vi "fg_ROI Management.vi"(0 "Dwell Time [us]":dbl, 1 "ROIs for deletion":i32[](array[numeric]), 2 "Laser Power %":dbl, 3 "Function":T5, 5 "Offsets cluster":T2, 7 "XYZ":T1 {"Apparent Frame Size" format="%#_6f"; "Original FOV (um)" format="%#_6f"; "Pixels per miniscan" format="%#_6f"; "Dwell Time per pixel" format="%#_6f"; "Resolution" format="%#_6f"; "ROI group ID" format="%#_6f"; "Laser Power (%)" format="%#_6f"; "Zoom" format="%#_6f"; "Frame Size" format="%#_6f"; "Number of lines" format="%#_6f"; "Composite ID" format="%#_6f"; "Angle (deg)" format="%#_6f"; "ROI Time (ns)" format="%#_6f"; "ROI ID" format="%#_6f"; "Pixels in ROI" format="%#_6f"; "ROI index" format="%#_6f"; "Z stop" format="%#_6f"; "Y stop" format="%#_6f"; "X stop" format="%#_6f"; "Z start" format="%#_6f"; "X start" format="%#_6f"; "Y start" format="%#_6f"}, 9 "ROI management Input cluster":T3, 11 "error in (no error)":errorcluster, 13 "ROI Setup Array Idx to modify":i32) -> (4 "ROI Setup":T1[](array[typedef]) {"Apparent Frame Size" format="%#_6f"; "Original FOV (um)" format="%#_6f"; "Pixels per miniscan" format="%#_6f"; "Dwell Time per pixel" format="%#_6f"; "Resolution" format="%#_6f"; "ROI group ID" format="%#_6f"; "Laser Power (%)" format="%#_6f"; "Zoom" format="%#_6f"; "Frame Size" format="%#_6f"; "Number of lines" format="%#_6f"; "Composite ID" format="%#_6f"; "Angle (deg)" format="%#_6f"; "ROI Time (ns)" format="%#_6f"; "ROI ID" format="%#_6f"; "Pixels in ROI" format="%#_6f"; "ROI index" format="%#_6f"; "Z stop" format="%#_6f"; "Y stop" format="%#_6f"; "X stop" format="%#_6f"; "Z start" format="%#_6f"; "X start" format="%#_6f"; "Y start" format="%#_6f"}, 6 "Number of ROI":i32, 8 "Total ROI time":dbl, 10 "Last composite ID":i32, 12 "Exceeded limit number of lines":bool, 14 "No lines left":bool, 15 "error out":errorcluster)   [LabVIEW 2020]
uses:
  Visualisation/Functional Imaging Viewer/Typedefs/ROI parameters data type.ctl
  Typedefs/ROI management FG states.ctl
  Typedefs/ROI management Input cluster.ctl
  Typedefs/ROI ID Enum.ctl
  Typedefs/Offsets cluster.ctl
  Global Variables/General Globals.vi
  ROI Entry screen/Globals/gl_ROI Entry UI globals.vi
panel:
  out "Number of lines left":i32
  in  "Reuse last composite ID":bool
  # "[zero based]"
  # "X Start\nY Start\nX Stop\nY Stop"
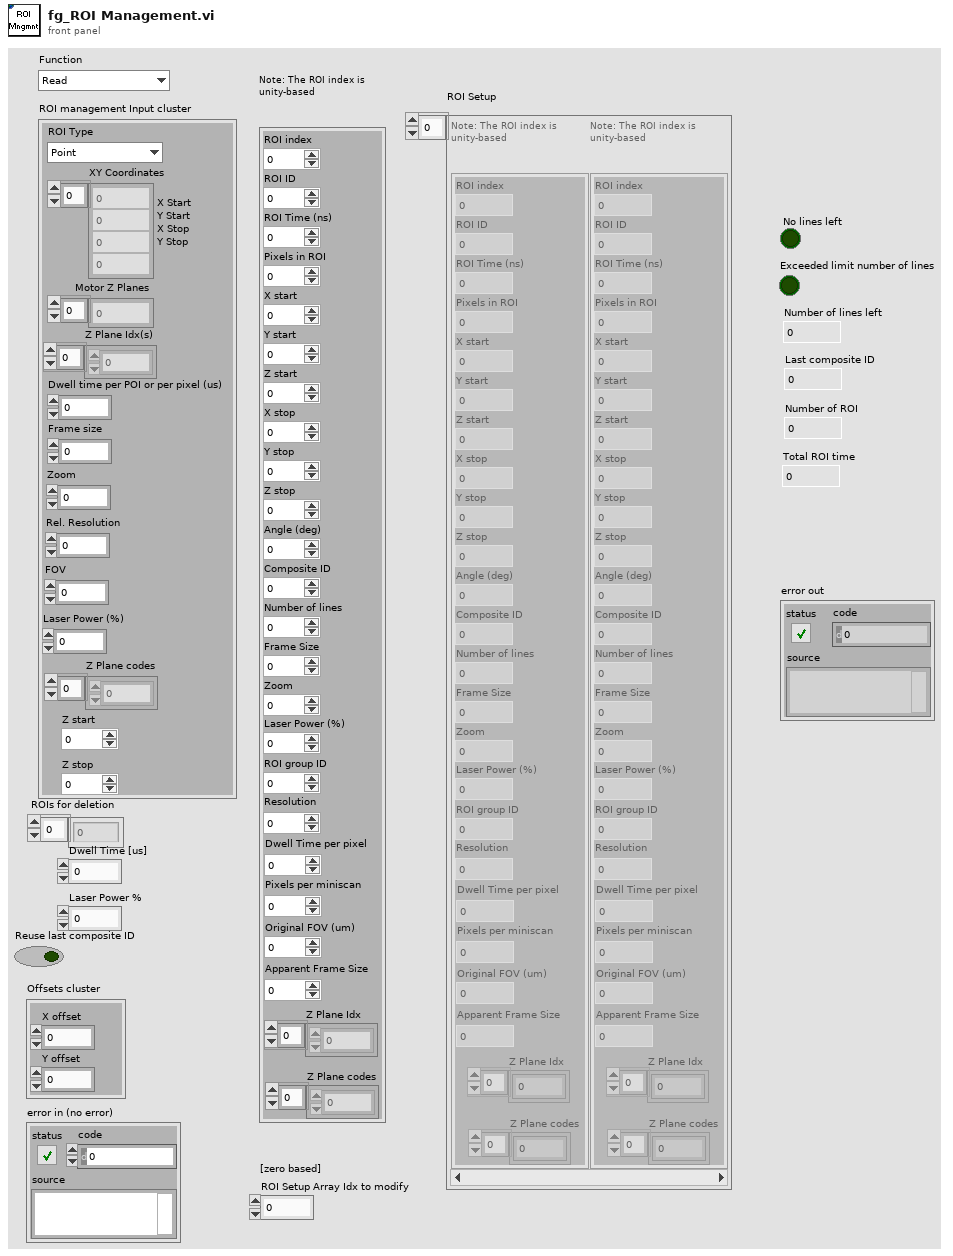
[diagram p1: front panel]
types:
  T1 = typedef "ROI parameters data type.ctl" = cluster{"ROI index":dbl, "ROI ID":dbl, "ROI Time (ns)":dbl, "Pixels in ROI":dbl, "X start":dbl, "Y start":dbl, "Z start":dbl, "X stop":dbl, "Y stop":dbl, "Z stop":dbl, "Angle (deg)":dbl, "Composite ID":dbl, "Number of lines":dbl, "Frame Size":dbl, "Zoom":dbl, "Laser Power (%)":dbl, "ROI group ID":dbl, "Resolution":dbl, "Dwell Time per pixel":dbl, "Pixels per miniscan":dbl, "Original FOV (um)":dbl, "Apparent Frame Size":dbl, "Z Plane Idx":i32[], "Z Plane codes":i32[]}
  T2 = typedef "Offsets cluster.ctl" = cluster{"X offset":i8, "Y offset":i8}
  T3 = typedef "ROI management Input cluster.ctl" = cluster{"ROI Type":T4, "XY Coordinates":i32[], "Motor Z Planes":dbl[], "Dwell time per POI or per pixel (us)":dbl, "Frame size":i32, "Zoom":dbl, "Rel. Resolution":dbl, "FOV":dbl, "Laser Power (%)":dbl, "Z Plane codes":u8[], "Z start":dbl, "Z stop":dbl, "Z Plane Idx(s)":i32[]}
  T4 = typedef "ROI ID Enum.ctl" = enum16{"Point", "MiniScan", "Comp. MiniScan", "Rectangle", "Comp. volume", "Arb. plane point", "None"}
  T5 = typedef "ROI management FG states.ctl" = enum16{"Read", "Write", "Write-from dataset", "Clear Last", "Clear All", "Delete ROI", "Update ROIs time", "Reload last ROI set", "Modify ROI Parameters", "Offset all ROI", "Offset visible ROI", "Modify Dwell Time", "Modify Laser Power"}
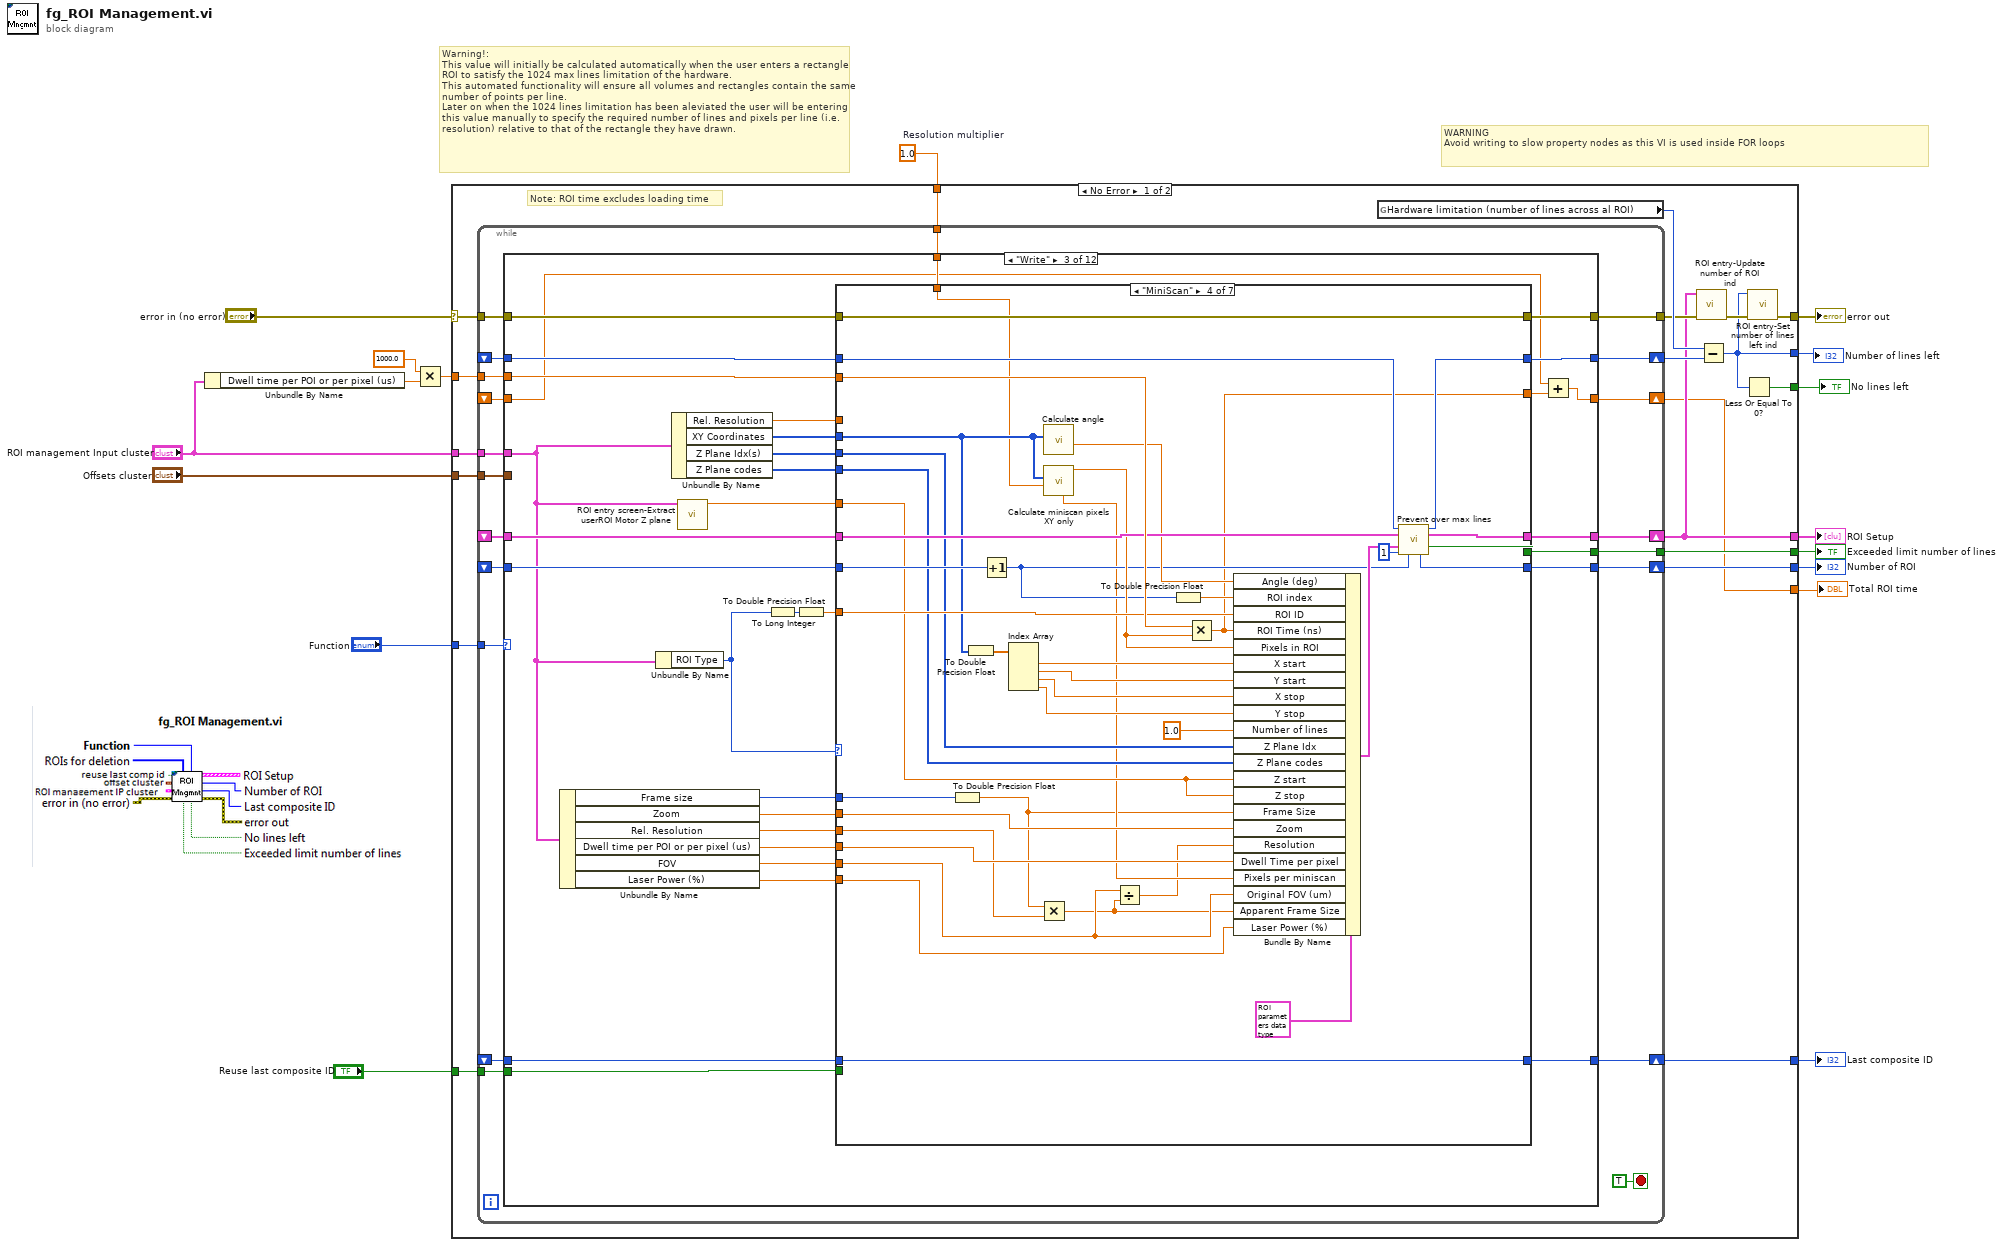
[diagram p0: block diagram]
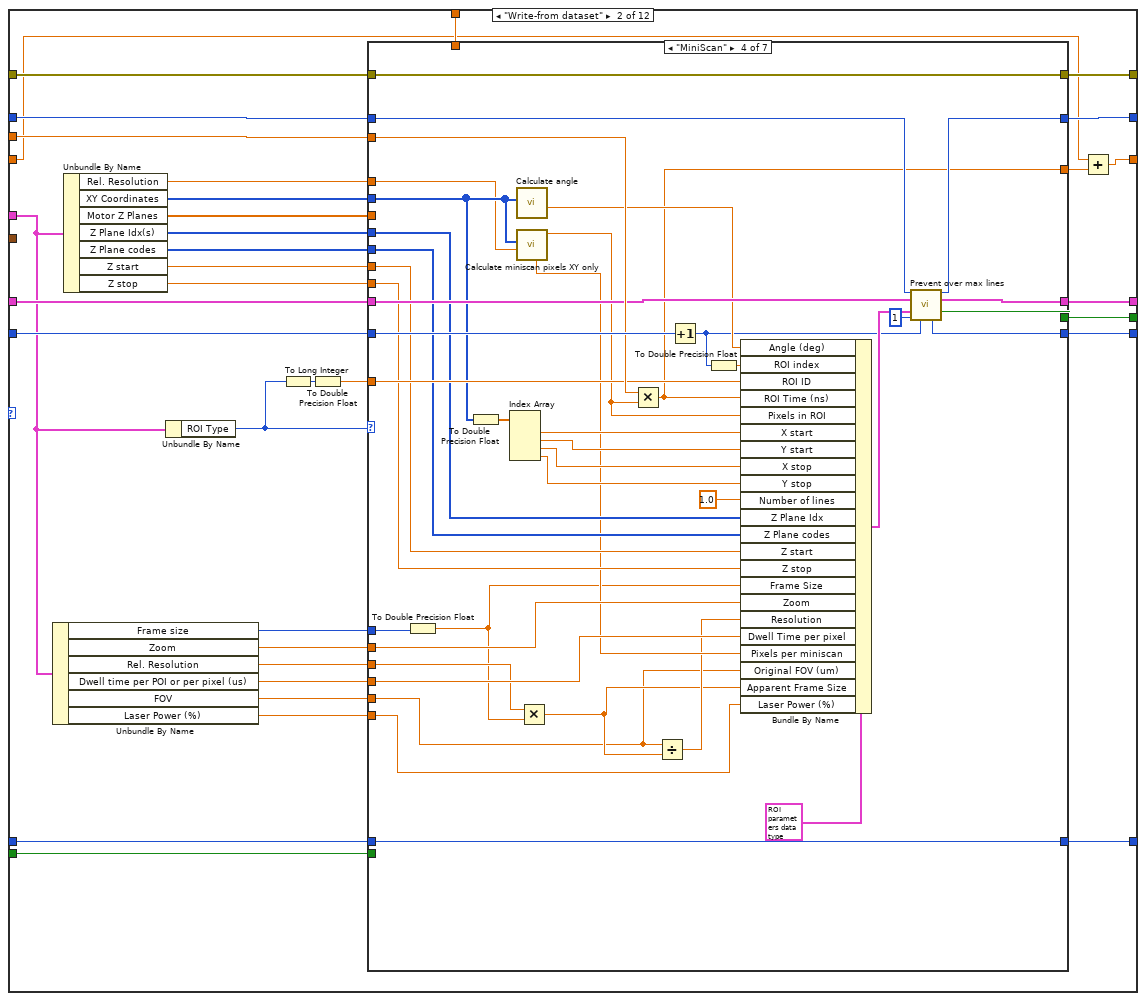
[diagram p3: hidden frame]
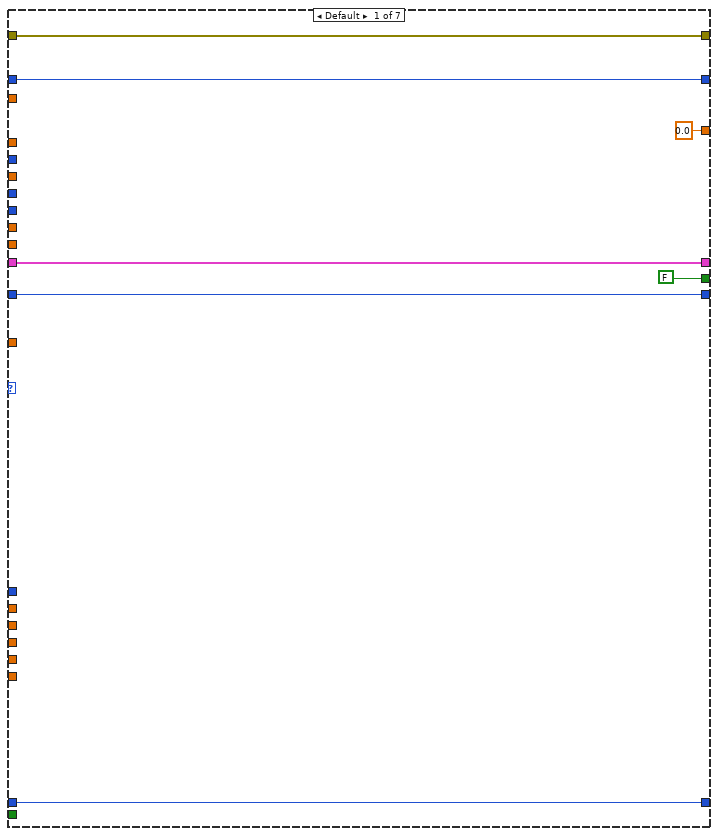
[diagram p4: hidden frame]
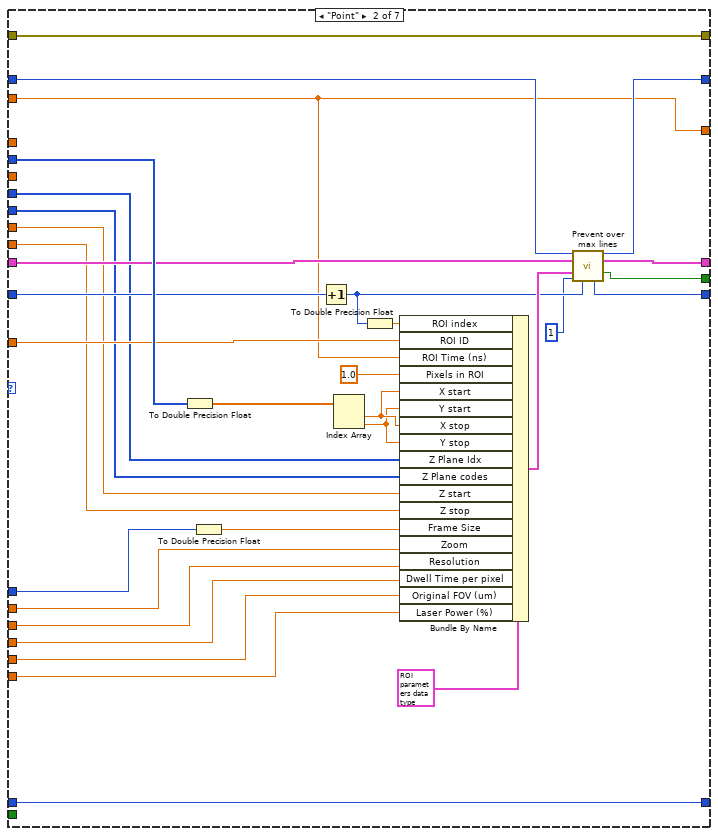
[diagram p5: hidden frame]
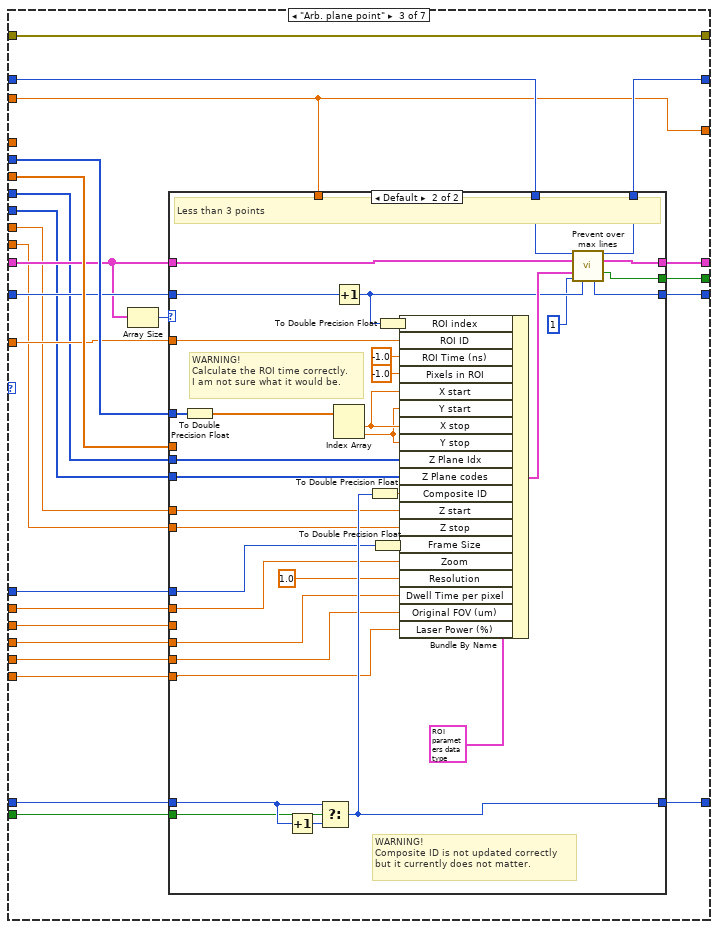
[diagram p6: hidden frame]
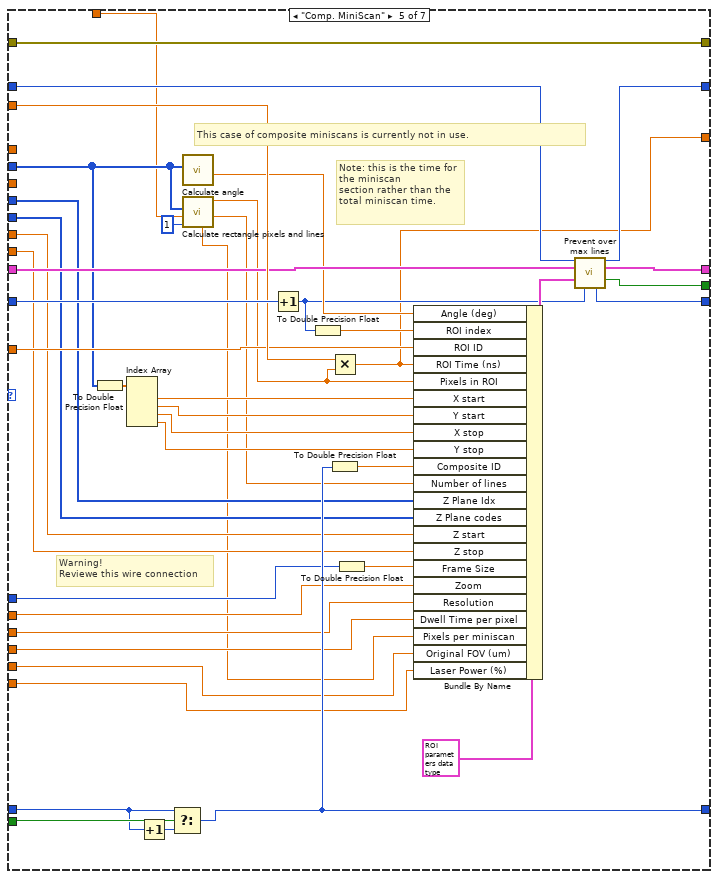
[diagram p8: hidden frame]
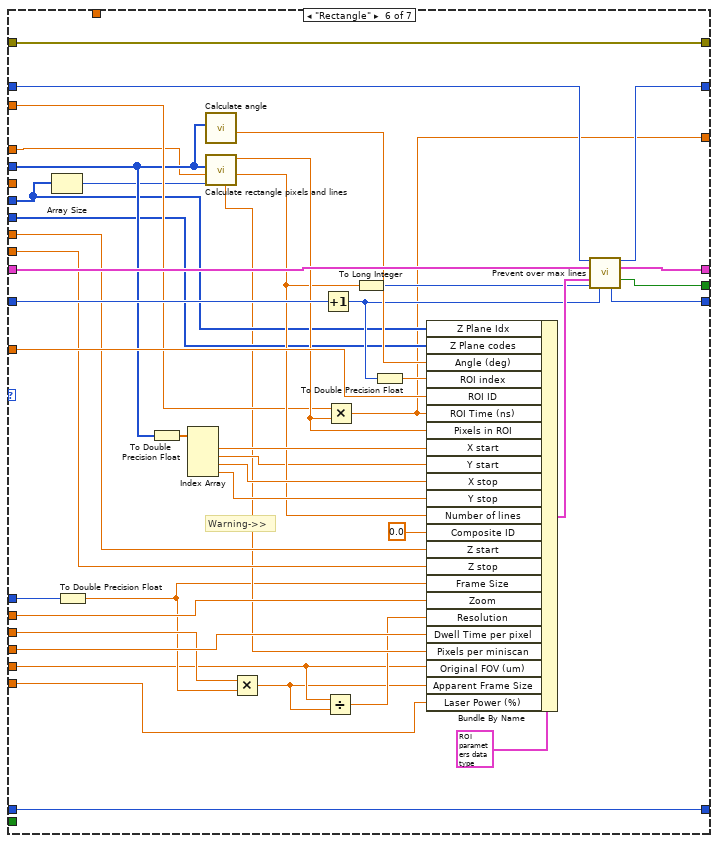
[diagram p9: hidden frame]
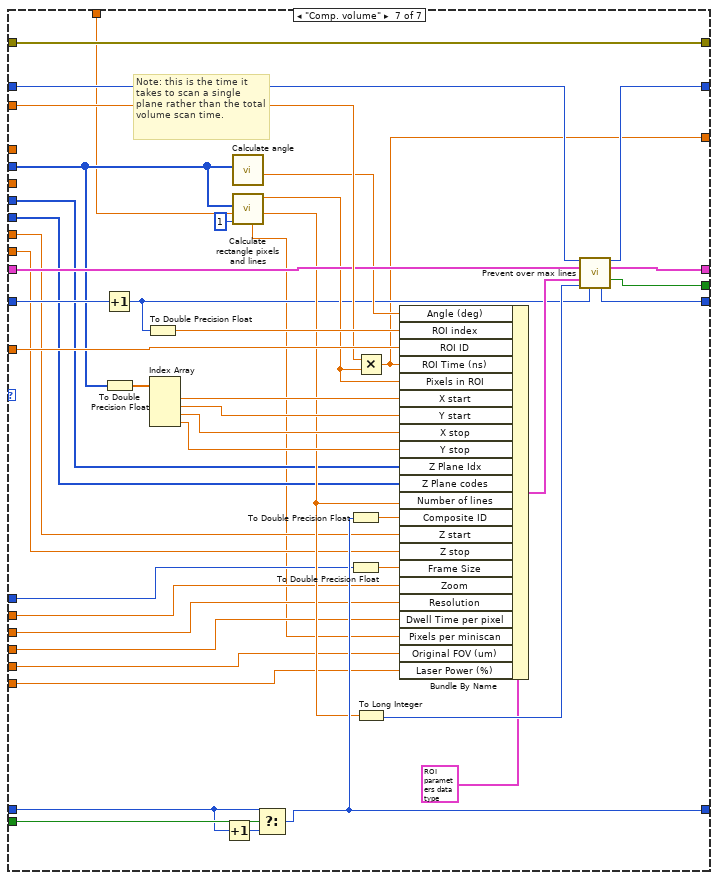
[diagram p10: hidden frame]
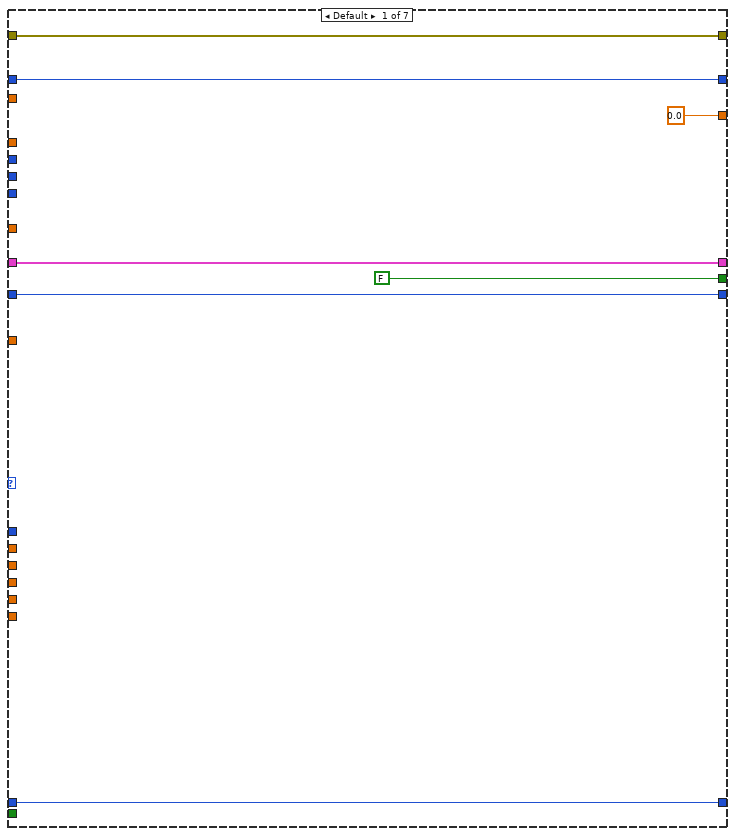
[diagram p11: hidden frame]
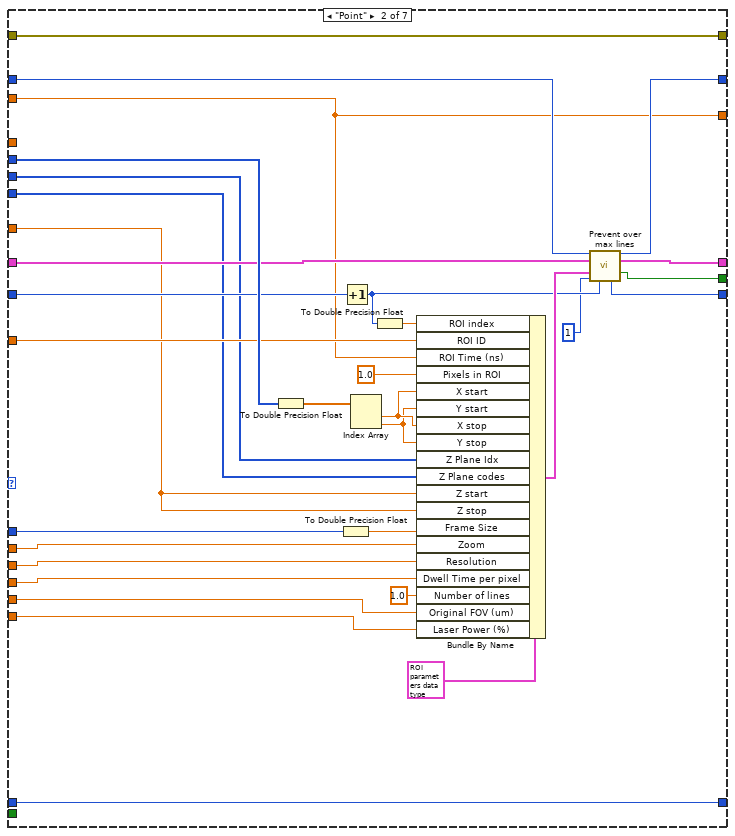
[diagram p12: hidden frame]
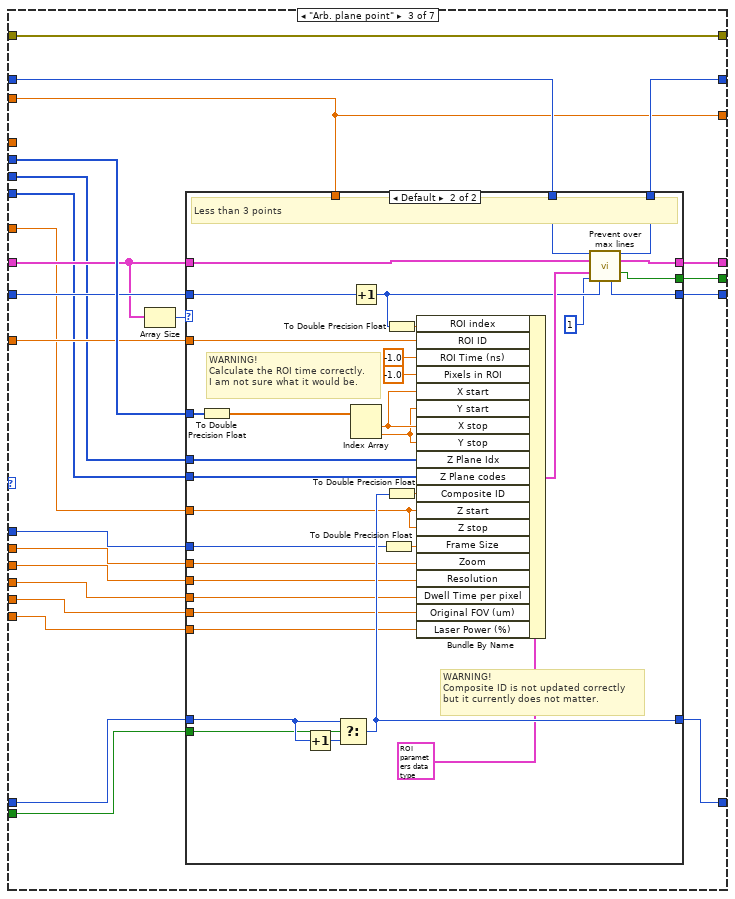
[diagram p13: hidden frame]
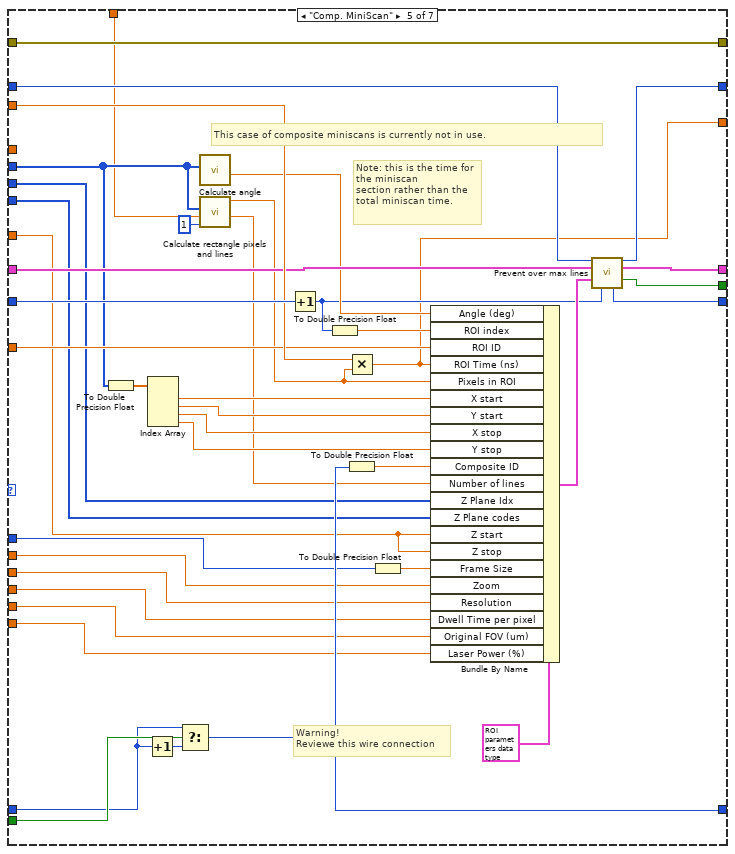
[diagram p15: hidden frame]
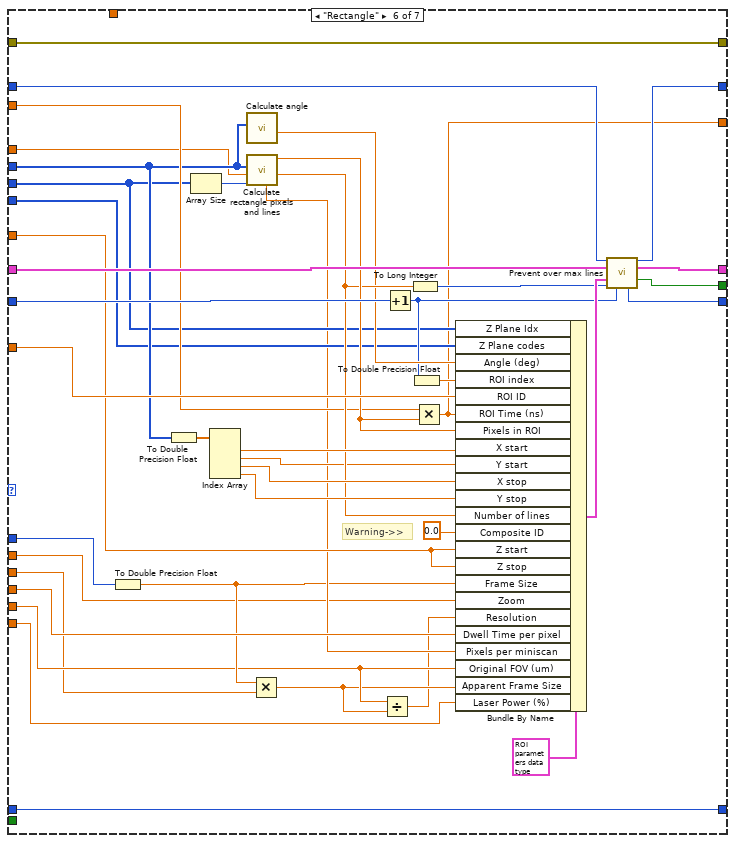
[diagram p16: hidden frame]
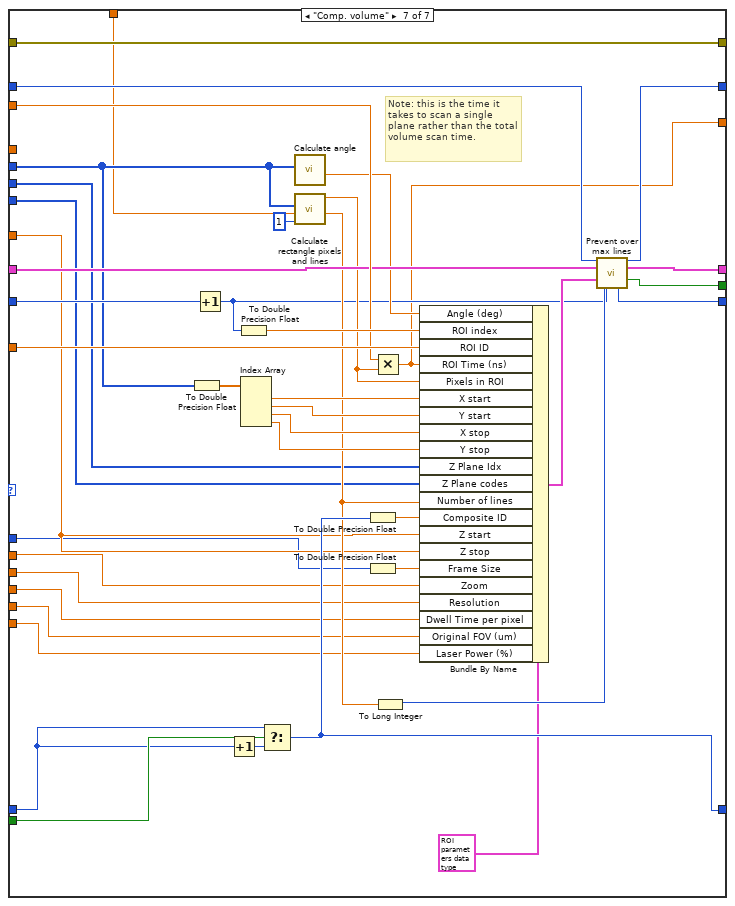
[diagram p17: hidden frame]
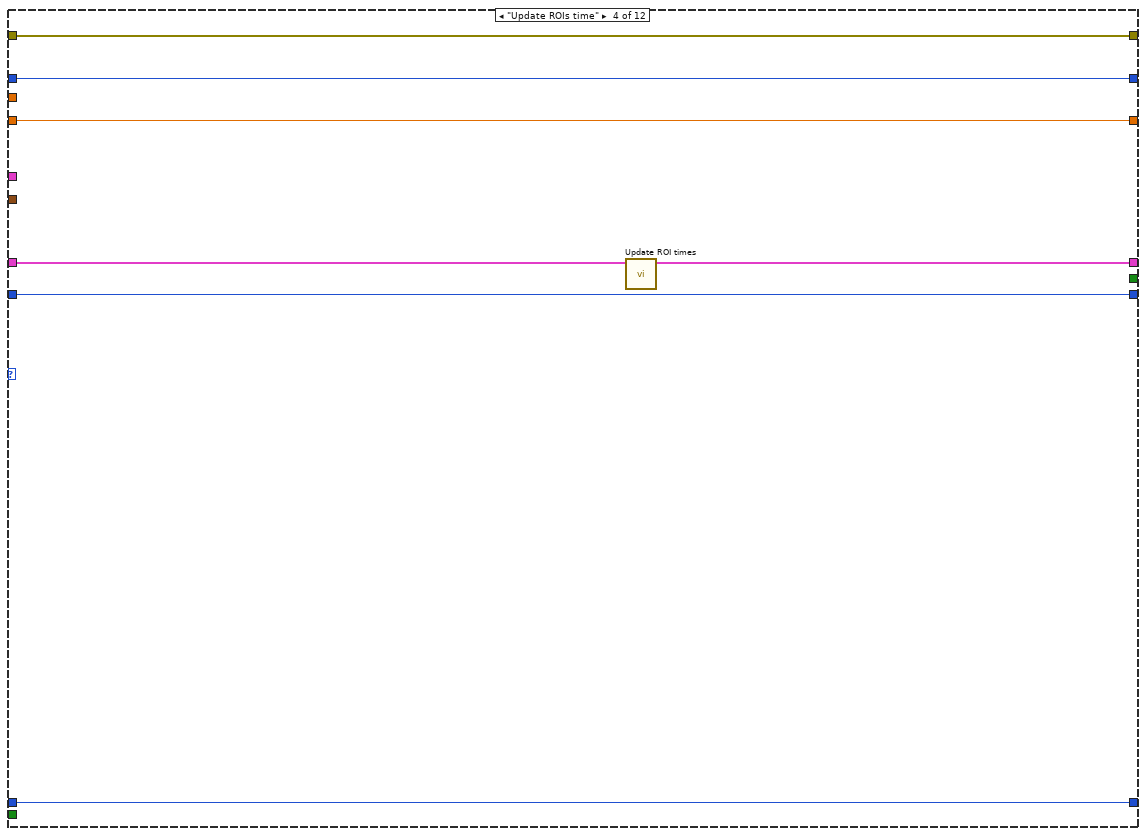
[diagram p18: hidden frame]
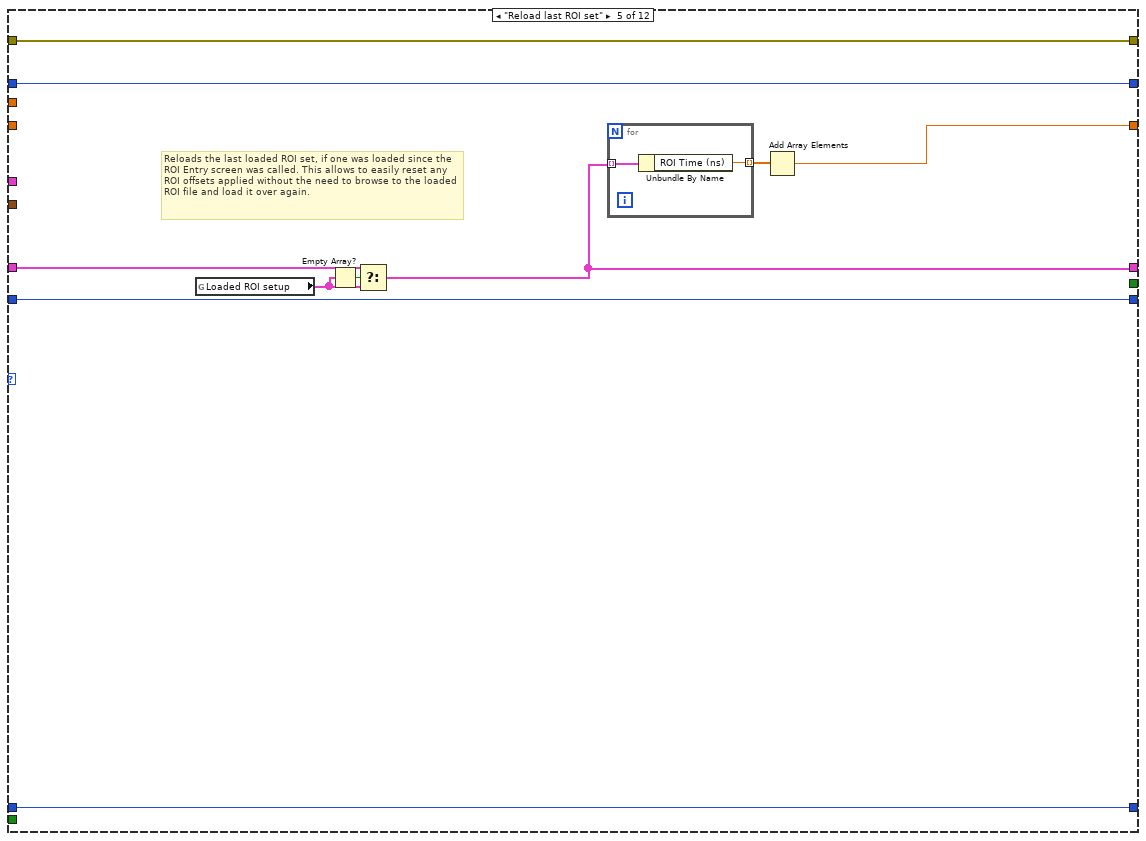
[diagram p19: hidden frame]
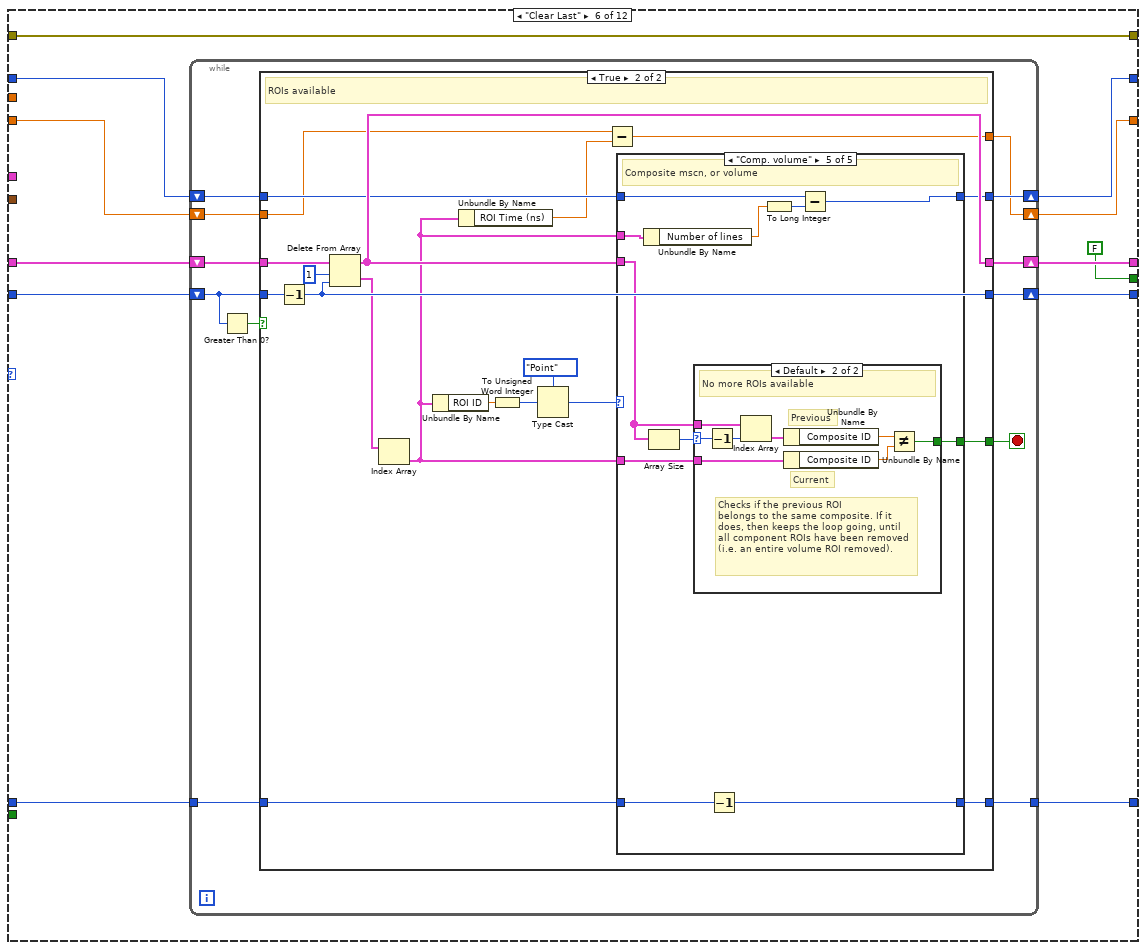
[diagram p20: hidden frame]
diagram:
  w7 = 1.0  # Resolution multiplier
  # "WARNING\nAvoid writing to slow property nodes as this VI is used inside FOR loops"
  # "Warning!:\nThis value will initially be calculated automatically when the user enters a rectangle ROI to satisfy the 1024 max lines limitation of the hardware.\nThis automated functionality will ensure all volumes and rectangles contain the same number of points per line.\nLater on when the 1024 lines limitation has been aleviated the user will be entering this value manually to specify the required number of lines and pixels per line (i.e. resolution) relative to that of the rectangle they have drawn."
  n1 = Unbundle By Name("ROI management Input cluster") -> ("Dwell time per POI or per pixel (us)"=w8:dbl)
  n2 = Multiply(x=1000.0, y=w8) -> (x*y=w13:dbl)
  n3 = case shown="No Error" "error in (no error)" {
    selector: "error in (no error)" -> [w36 w867]
    tunnel: [w22 w867] -> w14
    tunnel: [w24 _] -> w16
    tunnel: w13 -> [w35 _]
    tunnel: "Function" -> [w34 _]
    tunnel: [w33 _] -> w11
    tunnel: [w32 _] -> w10
    tunnel: "Reuse last composite ID" -> [w31 _]
    tunnel: "ROI management Input cluster" -> [w30 _]
    tunnel: w7 -> [w29 _]
    tunnel: [w20 _] -> w5
    tunnel: [w26 _] -> w4
    tunnel: "Offsets cluster" -> [w21 _]
    tunnel: [w19 _] -> w2
    tunnel: [w18 0.0 ("ROI Time (ns)o/p")] -> w1
    frame No Error {
      # "Note: ROI time excludes loading time"
      n4 = while {
        tunnel: w36 -> [w56]
        tunnel: [w55] -> w25
        shift-right: [w54] -> w24
        shift-left: _ -> [w52]
        tunnel: w35 -> [w53]
        shift-right: [w51] -> w33
        shift-left: _ -> [w50]
        tunnel: w34 -> [w49]
        shift-right: [w46] -> w32
        shift-left: _ -> [w47]
        tunnel: w31 -> [w45]
        tunnel: w30 -> [w44]
        shift-right: [w43] -> w28
        shift-left: _ -> [w42]
        tunnel: w29 -> [w41]
        tunnel: [w40] -> w26
        tunnel: w21 -> [w39]
        shift-right: [w38] -> w18
        shift-left: _ -> [w37]
        stop <- TRUE stop-if-true
        n5 = case shown="\"Write\"" w49 {
          selector: w49 -> [_ _ _ _ _ _ _ w798 _ _ _ _]
          tunnel: w56 -> [w60 w96 w403 w674 w685 w698 w795 w804 w809 w831 w842 w858]
          tunnel: [w60 w95 w402 w674 w685 w698 w795 w804 w809 w831 w842 w858] -> w55
          tunnel: [w62 w94 w401 w676 w679 w699 T1[] [] w799 w814 w825 w845 w860] -> w54
          tunnel: w53 -> [_ w93 w373 _ _ _ _ _ _ _ _ _]
          tunnel: w52 -> [w62 w92 w400 w672 w681 w694 _ w802 w815 w817 w847 w862]
          tunnel: [w61 w91 w399 w675 w686 w700 0 w805 w813 w818 w844 w859] -> w51
          tunnel: w50 -> [w61 w90 w398 w675 w686 w695 _ w805 _ w819 w844 w859]
          tunnel: w47 -> [w59 w86 w394 w671 w683 w697 _ w801 w808 w830 w841 w856]
          tunnel: [w59 w87 w395 w671 w683 w696 0 ("Last composite ID") w801 w808 w830 w841 w856] -> w46
          tunnel: w45 -> [_ w85 w393 _ _ _ _ _ _ _ _ _]
          tunnel: w44 -> [_ w81 w384 _ _ _ _ _ _ _ _ _]
          tunnel: [w58 w78 w388 w673 w684 w691 0 w803 w810 w820 w843 w857] -> w43
          tunnel: w42 -> [w58 w80 w390 w673 w684 w693 _ w803 w811 w821 w843 w857]
          tunnel: w41 -> [_ w79 w389 _ _ _ _ _ _ _ _ _]
          tunnel: [_ w77 w387 _ _ FALSE ("Exceeded 1024 lines") FALSE ("Exceeded 1024 lines") _ _ _ _ _] -> w40
          tunnel: w39 -> [_ _ _ _ _ _ _ w800 _ _ _ _]
          tunnel: [w57 w63 w375 w670 w677 w689 0.0 w797 w806 w826 w839 w855] -> w38
          tunnel: w37 -> [w57 w65 w372 w670 _ w690 _ w797 w807 w828 _ w855]
          frame "Read", Default {
          }
          frame "Write-from dataset" {
            n6 = Unbundle By Name(w81) -> ("Frame size"=w72:i32, "Zoom"=w71:dbl, "Rel. Resolution"=w70:dbl, "Dwell time per POI or per pixel (us)"=w69:dbl, "FOV"=w67:dbl, "Laser Power (%)"=w66:dbl)
            n7 = Unbundle By Name(w81) -> ("Rel. Resolution"=w68:dbl, "XY Coordinates"=w84:i32[], "Motor Z Planes"=w83:dbl[], "Z Plane Idx(s)"=w76:i32[], "Z Plane codes"=w75:u8[], "Z start"=w74:dbl, "Z stop"=w73:dbl)
            n8 = Unbundle By Name(w81) -> ("ROI Type"=w82:T4)
            n9 = To Long Integer(number=w82) -> (32bit integer=w89:i32)
            n10 = To Double Precision Float(number=w89) -> (double precision float=w88:dbl)
            n11 = case shown="\"MiniScan\"" w82 {
              tunnel: w84 -> [_ w134 w159 w225 w263 w308 w349]
              tunnel: w83 -> [_ _ w160 _ _ _ _]
              tunnel: w96 -> [w101 w135 w161 w241 w284 w327 w371]
              tunnel: [w101 w135 w161 w241 w284 w327 w371] -> w95
              tunnel: [w103 w125 w157 w229 w267 w319 w354] -> w94
              tunnel: w93 -> [_ w104 w136 w237 w280 w309 w362]
              tunnel: w92 -> [w103 w126 w153 w231 w269 w321 w356]
              tunnel: w90 -> [w102 w132 w158 w240 w283 w326 w370]
              tunnel: [w102 w119 w151 w220 w257 w303 w343] -> w91
              tunnel: w88 -> [_ w128 w147 w234 w275 w324 w364]
              tunnel: [w100 w127 w148 w233 w271 w322 w357] -> w87
              tunnel: w86 -> [w100 w127 w150 w233 w270 w322 w359]
              tunnel: w85 -> [_ _ w149 _ w272 _ w360]
              tunnel: [w99 w124 w156 w227 w266 w318 w353] -> w78
              tunnel: w80 -> [w99 w123 w155 w228 w265 w317 w352]
              tunnel: w79 -> [_ _ _ _ w260 _ w345]
              tunnel: [FALSE ("Exceeded 1024 lines") w122 w154 w226 w264 w316 w350] -> w77
              tunnel: w76 -> [_ w117 w146 w218 w255 w301 w341]
              tunnel: w75 -> [_ w118 w145 w219 w256 w302 w342]
              tunnel: w74 -> [_ w115 w144 w217 w254 w299 w339]
              tunnel: w73 -> [_ w114 w143 w216 w253 w298 w338]
              tunnel: w72 -> [_ w112 w142 w213 w250 w291 w336]
              tunnel: w71 -> [_ w111 w141 w212 w249 w297 w335]
              tunnel: w70 -> [_ w110 w140 w207 w248 w292 w334]
              tunnel: w69 -> [_ w109 w139 w211 w247 w296 w333]
              tunnel: w68 -> [_ _ _ w208 _ w293 _]
              tunnel: w67 -> [_ w107 w138 w203 w244 w288 w330]
              tunnel: w66 -> [_ w106 w137 w202 w243 w286 w329]
              tunnel: [0.0 w104 w136 w201 w242 w285 w328] -> w64
              frame Default {
              }
              frame "Point" {
                n12 = To Double Precision Float(number=w134) -> (double precision float=w130:dbl[])
                n13 = To Double Precision Float(number=w112) -> (double precision float=w113:dbl)
                n14 = Increment(x=w132) -> (x+1=w120:i32)
                n15 = Index Array(array=w130) -> (element #1=w131:dbl, element #2=w121:dbl)  [unwired: 2 in]
                n16 = To Double Precision Float(number=w120) -> (double precision float=w129:dbl)
                n17 = Bundle By Name(cluster=T1 {"ROI index"=0.0, "ROI ID"=0.0, "ROI Time (ns)"=0.0, "Pixels in ROI"=0.0, "X start"=0.0, "Y start"=0.0, "Z start"=0.0, "X stop"=0.0, "Y stop"=0.0, "Z stop"=0.0, "Angle (deg)"=0.0, "Composite ID"=0.0, "Number of lines"=0.0, "Frame Size"=0.0, "Zoom"=0.0, "Laser Power (%)"=0.0, "ROI group ID"=0.0, "Resolution"=0.0, "Dwell Time per pixel"=0.0, "Pixels per miniscan"=0.0, "Original FOV (um)"=0.0, "Apparent Frame Size"=0.0, "Z Plane Idx"=[], "Z Plane codes"=[]} ("X-Y-Z coordinates"), "ROI index"=w129, "ROI ID"=w128, "ROI Time (ns)"=w104, "Pixels in ROI"=1.0 ("#Pixels"), "X start"=w131, "Y start"=w121, "X stop"=w131, "Y stop"=w121, "Z Plane Idx"=w117, "Z Plane codes"=w118, "Z start"=w115, "Z stop"=w114, "Frame Size"=w113, "Zoom"=w111, "Resolution"=w110, "Dwell Time per pixel"=w109, "Original FOV (um)"=w107, "Laser Power (%)"=w106) -> (w133:T1)
                n18 = call "Prevent over max lines.vi"("Existing number of lines across all ROI"=w123, "Array in"=w126, "X-Y-Z coordinates"=w133, "New number of lines to be added (1)"=1, "Number of ROI"=w120) -> ("Resulting number of lines across all ROI"=w124:i32, "Array out"=w125:T1[], "Exceeded 1024 lines"=w122:bool, "Number of ROI"=w119:i32)  [unwired: 5 in, 2 out]
              }
              frame "Arb. plane point" {
                n19 = Array Size(array=w153) -> (size(s)=w152:i32)
                n20 = case shown="Default" w152 {
                  selector: w152 -> [w163 _]
                  tunnel: w160 -> [_ _]
                  tunnel: w159 -> [_ w200]
                  tunnel: w158 -> [_ w198]
                  tunnel: w136 -> [_ _]
                  tunnel: [w164 w193] -> w157
                  tunnel: [w165 w192] -> w156
                  tunnel: w155 -> [w165 w191]
                  tunnel: [_ w190] -> w154
                  tunnel: w153 -> [w164 w188]
                  tunnel: [w163 w179] -> w151
                  tunnel: w150 -> [w162 w186]
                  tunnel: w149 -> [_ w185]
                  tunnel: [w162 w183] -> w148
                  tunnel: w147 -> [_ w182]
                  tunnel: w146 -> [_ w177]
                  tunnel: w145 -> [_ w178]
                  tunnel: w144 -> [_ w175]
                  tunnel: w143 -> [_ w174]
                  tunnel: w142 -> [_ w171]
                  tunnel: w141 -> [_ w170]
                  tunnel: w140 -> [_ _]
                  tunnel: w139 -> [_ w169]
                  tunnel: w138 -> [_ w167]
                  tunnel: w137 -> [_ w166]
                  frame 3.. {
                    # "3 points (or more) already entered"
                  }
                  frame Default {
                    # "WARNING!\nComposite ID is not updated correctly\nbut it currently does not matter."
                    # "WARNING!\nCalculate the ROI time correctly.\nI am not sure what it would be."
                    # "Less than 3 points"
                    n21 = To Double Precision Float(number=w200) -> (double precision float=w195:dbl[])
                    n22 = Increment(x=w186) -> (x+1=w187:i32)
                    n23 = Select(t=w186, s=w185, f=w187) -> (s? t:f=w183:i32)
                    n24 = Increment(x=w198) -> (x+1=w180:i32)
                    n25 = Index Array(array=w195) -> (element #1=w196:dbl, element #2=w189:dbl)  [unwired: 2 in]
                    n26 = To Double Precision Float(number=w183) -> (double precision float=w184:dbl)
                    n27 = To Double Precision Float(number=w171) -> (double precision float=w172:dbl)
                    n28 = To Double Precision Float(number=w180) -> (double precision float=w194:dbl)
                    n29 = Bundle By Name(cluster=T1 {"ROI index"=0.0, "ROI ID"=0.0, "ROI Time (ns)"=0.0, "Pixels in ROI"=0.0, "X start"=0.0, "Y start"=0.0, "Z start"=0.0, "X stop"=0.0, "Y stop"=0.0, "Z stop"=0.0, "Angle (deg)"=0.0, "Composite ID"=0.0, "Number of lines"=0.0, "Frame Size"=0.0, "Zoom"=0.0, "Laser Power (%)"=0.0, "ROI group ID"=0.0, "Resolution"=0.0, "Dwell Time per pixel"=0.0, "Pixels per miniscan"=0.0, "Original FOV (um)"=0.0, "Apparent Frame Size"=0.0, "Z Plane Idx"=[], "Z Plane codes"=[]} ("X-Y-Z coordinates"), "ROI index"=w194, "ROI ID"=w182, "ROI Time (ns)"=-1.0, "Pixels in ROI"=-1.0 ("#Pixels"), "X start"=w196, "Y start"=w189, "X stop"=w196, "Y stop"=w189, "Z Plane Idx"=w177, "Z Plane codes"=w178, "Composite ID"=w184, "Z start"=w175, "Z stop"=w174, "Frame Size"=w172, "Zoom"=w170, "Resolution"=1.0, "Dwell Time per pixel"=w169, "Original FOV (um)"=w167, "Laser Power (%)"=w166) -> (w199:T1)
                    n30 = call "Prevent over max lines.vi"("Existing number of lines across all ROI"=w191, "Array in"=w188, "X-Y-Z coordinates"=w199, "New number of lines to be added (1)"=1, "Number of ROI"=w180) -> ("Resulting number of lines across all ROI"=w192:i32, "Array out"=w193:T1[], "Exceeded 1024 lines"=w190:bool, "Number of ROI"=w179:i32)  [unwired: 5 in, 2 out]
                  }
                }
              }
              frame "MiniScan" {
                n31 = To Double Precision Float(number=w213) -> (double precision float=w206:dbl)
                n32 = To Double Precision Float(number=w225) -> (double precision float=w238:dbl[])
                n33 = Index Array(array=w238) -> (element #1=w222:dbl, element #2=w239:dbl, element #3=w232:dbl, element #4=w235:dbl)  [unwired: 4 in]
                n34 = call "Calculate angle.vi"("XY Coordinates"=w225) -> ("Angle (deg)"=w223:dbl)  [unwired: 10 in]
                n35 = call "Calculate miniscan pixels XY only.vi"("Resolution multiplier"=w208, "XY Coordinates (zero based)"=w225) -> ("Pixels in ROI"=w224:dbl, "X pixels"=w209:dbl)  [unwired: 7 in, 1 out]
                n36 = Multiply(x=w207, y=w206) -> (x*y=w204:dbl)
                n37 = Multiply(x=w237, y=w224) -> (x*y=w201:dbl)
                n38 = Divide(x=w203, y=w204) -> (x/y=w205:dbl)
                n39 = Increment(x=w240) -> (x+1=w221:i32)
                n40 = To Double Precision Float(number=w221) -> (double precision float=w236:dbl)
                n41 = Bundle By Name(cluster=T1 {"ROI index"=0.0, "ROI ID"=0.0, "ROI Time (ns)"=0.0, "Pixels in ROI"=0.0, "X start"=0.0, "Y start"=0.0, "Z start"=0.0, "X stop"=0.0, "Y stop"=0.0, "Z stop"=0.0, "Angle (deg)"=0.0, "Composite ID"=0.0, "Number of lines"=0.0, "Frame Size"=0.0, "Zoom"=0.0, "Laser Power (%)"=0.0, "ROI group ID"=0.0, "Resolution"=0.0, "Dwell Time per pixel"=0.0, "Pixels per miniscan"=0.0, "Original FOV (um)"=0.0, "Apparent Frame Size"=0.0, "Z Plane Idx"=[], "Z Plane codes"=[]} ("X-Y-Z coordinates"), "Angle (deg)"=w223, "ROI index"=w236, "ROI ID"=w234, "ROI Time (ns)"=w201, "Pixels in ROI"=w224, "X start"=w222, "Y start"=w239, "X stop"=w232, "Y stop"=w235, "Number of lines"=1.0, "Z Plane Idx"=w218, "Z Plane codes"=w219, "Z start"=w217, "Z stop"=w216, "Frame Size"=w206, "Zoom"=w212, "Resolution"=w205, "Dwell Time per pixel"=w211, "Pixels per miniscan"=w209, "Original FOV (um)"=w203, "Apparent Frame Size"=w204, "Laser Power (%)"=w202) -> (w230:T1)
                n42 = call "Prevent over max lines.vi"("Existing number of lines across all ROI"=w228, "Array in"=w231, "X-Y-Z coordinates"=w230, "New number of lines to be added (1)"=1, "Number of ROI"=w221) -> ("Resulting number of lines across all ROI"=w227:i32, "Array out"=w229:T1[], "Exceeded 1024 lines"=w226:bool, "Number of ROI"=w220:i32)  [unwired: 5 in, 2 out]
              }
              frame "Comp. MiniScan" {
                # "This case of composite miniscans is currently not in use."
                # "Warning!\nReviewe this wire connection"
                # "Note: this is the time for the miniscan\nsection rather than the total miniscan time."
                n43 = To Double Precision Float(number=w263) -> (double precision float=w281:dbl[])
                n44 = Index Array(array=w281) -> (element #1=w278:dbl, element #2=w282:dbl, element #3=w277:dbl, element #4=w276:dbl)  [unwired: 4 in]
                n45 = Increment(x=w270) -> (x+1=w273:i32)
                n46 = Select(t=w270, s=w272, f=w273) -> (s? t:f=w271:i32)
                n47 = call "Calculate angle.vi"("XY Coordinates"=w263) -> ("Angle (deg)"=w261:dbl)  [unwired: 10 in]
                n48 = call "Calculate rectangle pixels and lines.vi"("No of Z planes"=1, "Resolution multiplier"=w260, "XY Coordinates (zero based)"=w263) -> ("Number of lines (scaled)"=w259:dbl, "Pixels in ROI"=w262:dbl, "X pixels"=w245:dbl)  [unwired: 6 in]
                n49 = Increment(x=w283) -> (x+1=w258:i32)
                n50 = To Double Precision Float(number=w258) -> (double precision float=w279:dbl)
                n51 = Multiply(x=w280, y=w262) -> (x*y=w242:dbl)
                n52 = To Double Precision Float(number=w271) -> (double precision float=w274:dbl)
                n53 = To Double Precision Float(number=w250) -> (double precision float=w251:dbl)
                n54 = Bundle By Name(cluster=T1 {"ROI index"=0.0, "ROI ID"=0.0, "ROI Time (ns)"=0.0, "Pixels in ROI"=0.0, "X start"=0.0, "Y start"=0.0, "Z start"=0.0, "X stop"=0.0, "Y stop"=0.0, "Z stop"=0.0, "Angle (deg)"=0.0, "Composite ID"=0.0, "Number of lines"=0.0, "Frame Size"=0.0, "Zoom"=0.0, "Laser Power (%)"=0.0, "ROI group ID"=0.0, "Resolution"=0.0, "Dwell Time per pixel"=0.0, "Pixels per miniscan"=0.0, "Original FOV (um)"=0.0, "Apparent Frame Size"=0.0, "Z Plane Idx"=[], "Z Plane codes"=[]} ("X-Y-Z coordinates"), "Angle (deg)"=w261, "ROI index"=w279, "ROI ID"=w275, "ROI Time (ns)"=w242, "Pixels in ROI"=w262, "X start"=w278, "Y start"=w282, "X stop"=w277, "Y stop"=w276, "Composite ID"=w274, "Number of lines"=w259, "Z Plane Idx"=w255, "Z Plane codes"=w256, "Z start"=w254, "Z stop"=w253, "Frame Size"=w251, "Zoom"=w249, "Resolution"=w248, "Dwell Time per pixel"=w247, "Pixels per miniscan"=w245, "Original FOV (um)"=w244, "Laser Power (%)"=w243) -> (w268:T1)
                n55 = call "Prevent over max lines.vi"("Existing number of lines across all ROI"=w265, "Array in"=w269, "X-Y-Z coordinates"=w268, "Number of ROI"=w258) -> ("Resulting number of lines across all ROI"=w266:i32, "Array out"=w267:T1[], "Exceeded 1024 lines"=w264:bool, "Number of ROI"=w257:i32)  [unwired: 6 in, 2 out]
              }
              frame "Rectangle" {
                # "Warning->>"
                n56 = Array Size(array=w301) -> (size(s)=w300:i32)
                n57 = To Double Precision Float(number=w291) -> (double precision float=w290:dbl)
                n58 = To Double Precision Float(number=w308) -> (double precision float=w325:dbl[])
                n59 = Index Array(array=w325) -> (element #1=w315:dbl, element #2=w310:dbl, element #3=w314:dbl, element #4=w313:dbl)  [unwired: 4 in]
                n60 = call "Calculate angle.vi"("XY Coordinates"=w308) -> ("Angle (deg)"=w307:dbl)  [unwired: 10 in]
                n61 = call "Calculate rectangle pixels and lines.vi"("No of Z planes"=w300, "Resolution multiplier"=w293, "XY Coordinates (zero based)"=w308) -> ("Number of lines (scaled)"=w311:dbl, "Pixels in ROI"=w312:dbl, "X pixels"=w294:dbl)  [unwired: 6 in]
                n62 = Multiply(x=w292, y=w290) -> (x*y=w287:dbl)
                n63 = Increment(x=w326) -> (x+1=w304:i32)
                n64 = Divide(x=w288, y=w287) -> (x/y=w289:dbl)
                n65 = Multiply(x=w309, y=w312) -> (x*y=w285:dbl)
                n66 = To Long Integer(number=w311) -> (32bit integer=w305:i32)
                n67 = To Double Precision Float(number=w304) -> (double precision float=w323:dbl)
                n68 = Bundle By Name(cluster=T1 {"ROI index"=0.0, "ROI ID"=0.0, "ROI Time (ns)"=0.0, "Pixels in ROI"=0.0, "X start"=0.0, "Y start"=0.0, "Z start"=0.0, "X stop"=0.0, "Y stop"=0.0, "Z stop"=0.0, "Angle (deg)"=0.0, "Composite ID"=0.0, "Number of lines"=0.0, "Frame Size"=0.0, "Zoom"=0.0, "Laser Power (%)"=0.0, "ROI group ID"=0.0, "Resolution"=0.0, "Dwell Time per pixel"=0.0, "Pixels per miniscan"=0.0, "Original FOV (um)"=0.0, "Apparent Frame Size"=0.0, "Z Plane Idx"=[], "Z Plane codes"=[]} ("X-Y-Z coordinates"), "Z Plane Idx"=w301, "Z Plane codes"=w302, "Angle (deg)"=w307, "ROI index"=w323, "ROI ID"=w324, "ROI Time (ns)"=w285, "Pixels in ROI"=w312, "X start"=w315, "Y start"=w310, "X stop"=w314, "Y stop"=w313, "Number of lines"=w311, "Composite ID"=0.0, "Z start"=w299, "Z stop"=w298, "Frame Size"=w290, "Zoom"=w297, "Resolution"=w289, "Dwell Time per pixel"=w296, "Pixels per miniscan"=w294, "Original FOV (um)"=w288, "Apparent Frame Size"=w287, "Laser Power (%)"=w286) -> (w320:T1)
                n69 = call "Prevent over max lines.vi"("Existing number of lines across all ROI"=w317, "Array in"=w321, "X-Y-Z coordinates"=w320, "New number of lines to be added (1)"=w305, "Number of ROI"=w304) -> ("Resulting number of lines across all ROI"=w318:i32, "Array out"=w319:T1[], "Exceeded 1024 lines"=w316:bool, "Number of ROI"=w303:i32)  [unwired: 5 in, 2 out]
              }
              frame "Comp. volume" {
                # "Note: this is the time it takes to scan a single plane rather than the total volume scan time."
                n70 = Increment(x=w370) -> (x+1=w344:i32)
                n71 = To Double Precision Float(number=w349) -> (double precision float=w365:dbl[])
                n72 = To Double Precision Float(number=w344) -> (double precision float=w363:dbl)
                n73 = Index Array(array=w365) -> (element #1=w366:dbl, element #2=w369:dbl, element #3=w368:dbl, element #4=w367:dbl)  [unwired: 4 in]
                n74 = Increment(x=w359) -> (x+1=w358:i32)
                n75 = call "Calculate angle.vi"("XY Coordinates"=w349) -> ("Angle (deg)"=w348:dbl)  [unwired: 10 in]
                n76 = call "Calculate rectangle pixels and lines.vi"("No of Z planes"=1, "Resolution multiplier"=w345, "XY Coordinates (zero based)"=w349) -> ("Number of lines (scaled)"=w346:dbl, "Pixels in ROI"=w347:dbl, "X pixels"=w331:dbl)  [unwired: 6 in]
                n77 = Select(t=w359, s=w360, f=w358) -> (s? t:f=w357:i32)
                n78 = To Double Precision Float(number=w357) -> (double precision float=w361:dbl)
                n79 = To Double Precision Float(number=w336) -> (double precision float=w337:dbl)
                n80 = Multiply(x=w362, y=w347) -> (x*y=w328:dbl)
                n81 = To Long Integer(number=w346) -> (32bit integer=w351:i32)
                n82 = Bundle By Name(cluster=T1 {"ROI index"=0.0, "ROI ID"=0.0, "ROI Time (ns)"=0.0, "Pixels in ROI"=0.0, "X start"=0.0, "Y start"=0.0, "Z start"=0.0, "X stop"=0.0, "Y stop"=0.0, "Z stop"=0.0, "Angle (deg)"=0.0, "Composite ID"=0.0, "Number of lines"=0.0, "Frame Size"=0.0, "Zoom"=0.0, "Laser Power (%)"=0.0, "ROI group ID"=0.0, "Resolution"=0.0, "Dwell Time per pixel"=0.0, "Pixels per miniscan"=0.0, "Original FOV (um)"=0.0, "Apparent Frame Size"=0.0, "Z Plane Idx"=[], "Z Plane codes"=[]} ("X-Y-Z coordinates"), "Angle (deg)"=w348, "ROI index"=w363, "ROI ID"=w364, "ROI Time (ns)"=w328, "Pixels in ROI"=w347, "X start"=w366, "Y start"=w369, "X stop"=w368, "Y stop"=w367, "Z Plane Idx"=w341, "Z Plane codes"=w342, "Number of lines"=w346, "Composite ID"=w361, "Z start"=w339, "Z stop"=w338, "Frame Size"=w337, "Zoom"=w335, "Resolution"=w334, "Dwell Time per pixel"=w333, "Pixels per miniscan"=w331, "Original FOV (um)"=w330, "Laser Power (%)"=w329) -> (w355:T1)
                n83 = call "Prevent over max lines.vi"("Existing number of lines across all ROI"=w352, "Array in"=w356, "X-Y-Z coordinates"=w355, "New number of lines to be added (1)"=w351, "Number of ROI"=w344) -> ("Resulting number of lines across all ROI"=w353:i32, "Array out"=w354:T1[], "Exceeded 1024 lines"=w350:bool, "Number of ROI"=w343:i32)  [unwired: 5 in, 2 out]
              }
            }
            n84 = Add(x=w65, y=w64) -> (x+y=w63:dbl)
          }
          frame "Write" {
            n85 = Unbundle By Name(w384) -> ("Frame size"=w382:i32, "Zoom"=w381:dbl, "Rel. Resolution"=w380:dbl, "Dwell time per POI or per pixel (us)"=w379:dbl, "FOV"=w377:dbl, "Laser Power (%)"=w376:dbl)
            n86 = Unbundle By Name(w384) -> ("ROI Type"=w391:T4)
            n87 = Unbundle By Name(w384) -> ("Rel. Resolution"=w378:dbl, "XY Coordinates"=w392:i32[], "Z Plane Idx(s)"=w386:i32[], "Z Plane codes"=w385:u8[])
            n88 = call "ROI entry screen-Extract userROI Motor Z plane.vi"("ROI management Input cluster"=w384) -> ("Motor Z plane"=w383:dbl)  [unwired: 10 in]
            n89 = To Long Integer(number=w391) -> (32bit integer=w397:i32)
            n90 = To Double Precision Float(number=w397) -> (double precision float=w396:dbl)
            n91 = case shown="\"MiniScan\"" w391 {
              tunnel: w392 -> [_ w441 w465 w528 w564 w608 w647]
              tunnel: w403 -> [w408 w442 w466 w544 w585 w627 w669]
              tunnel: [w408 w442 w466 w544 w585 w627 w669] -> w402
              tunnel: [w410 w431 w463 w532 w568 w619 w652] -> w401
              tunnel: w373 -> [_ w411 w443 w540 w581 w609 w660]
              tunnel: w400 -> [w410 w432 w459 w534 w570 w621 w654]
              tunnel: w398 -> [w409 w439 w464 w543 w584 w626 w668]
              tunnel: [w409 w425 w457 w522 w558 w603 w641] -> w399
              tunnel: w396 -> [_ w434 w453 w537 w576 w624 w662]
              tunnel: [w407 w433 w454 w536 w572 w622 w655] -> w395
              tunnel: w394 -> [w407 w433 w456 w536 w571 w622 w657]
              tunnel: w393 -> [_ _ w455 _ w573 _ w658]
              tunnel: [w406 w430 w462 w530 w567 w618 w651] -> w388
              tunnel: w390 -> [w406 w429 w461 w531 w566 w617 w650]
              tunnel: w389 -> [_ _ _ w524 w561 _ w643]
              tunnel: [FALSE ("Exceeded 1024 lines") w428 w460 w529 w565 w616 w648] -> w387
              tunnel: w386 -> [_ w423 w452 w520 w556 w601 w639]
              tunnel: w385 -> [_ w424 w451 w521 w557 w602 w640]
              tunnel: w383 -> [_ w421 w450 w517 w554 w599 w637]
              tunnel: w382 -> [_ w420 w449 w516 w552 w594 w634]
              tunnel: w381 -> [_ w418 w448 w515 w551 w592 w633]
              tunnel: w380 -> [_ w417 w447 w510 w550 w588 w632]
              tunnel: w379 -> [_ w416 w446 w514 w549 w597 w631]
              tunnel: w378 -> [_ _ _ _ _ w595 _]
              tunnel: w377 -> [_ w413 w445 w508 w547 w591 w630]
              tunnel: w376 -> [_ w412 w444 w506 w546 w587 w629]
              tunnel: [0.0 w411 w443 w505 w545 w586 w628] -> w374
              frame Default {
              }
              frame "Point" {
                n92 = To Double Precision Float(number=w441) -> (double precision float=w436:dbl[])
                n93 = To Double Precision Float(number=w420) -> (double precision float=w419:dbl)
                n94 = Increment(x=w439) -> (x+1=w426:i32)
                n95 = Index Array(array=w436) -> (element #1=w437:dbl, element #2=w427:dbl)  [unwired: 2 in]
                n96 = To Double Precision Float(number=w426) -> (double precision float=w435:dbl)
                n97 = Bundle By Name(cluster=T1 {"ROI index"=0.0, "ROI ID"=0.0, "ROI Time (ns)"=0.0, "Pixels in ROI"=0.0, "X start"=0.0, "Y start"=0.0, "Z start"=0.0, "X stop"=0.0, "Y stop"=0.0, "Z stop"=0.0, "Angle (deg)"=0.0, "Composite ID"=0.0, "Number of lines"=0.0, "Frame Size"=0.0, "Zoom"=0.0, "Laser Power (%)"=0.0, "ROI group ID"=0.0, "Resolution"=0.0, "Dwell Time per pixel"=0.0, "Pixels per miniscan"=0.0, "Original FOV (um)"=0.0, "Apparent Frame Size"=0.0, "Z Plane Idx"=[], "Z Plane codes"=[]} ("X-Y-Z coordinates"), "ROI index"=w435, "ROI ID"=w434, "ROI Time (ns)"=w411, "Pixels in ROI"=1.0 ("#Pixels"), "X start"=w437, "Y start"=w427, "X stop"=w437, "Y stop"=w427, "Z Plane Idx"=w423, "Z Plane codes"=w424, "Z start"=w421, "Z stop"=w421, "Frame Size"=w419, "Zoom"=w418, "Resolution"=w417, "Dwell Time per pixel"=w416, "Number of lines"=1.0, "Original FOV (um)"=w413, "Laser Power (%)"=w412) -> (w440:T1)
                n98 = call "Prevent over max lines.vi"("Existing number of lines across all ROI"=w429, "Array in"=w432, "X-Y-Z coordinates"=w440, "New number of lines to be added (1)"=1, "Number of ROI"=w426) -> ("Resulting number of lines across all ROI"=w430:i32, "Array out"=w431:T1[], "Exceeded 1024 lines"=w428:bool, "Number of ROI"=w425:i32)  [unwired: 5 in, 2 out]
              }
              frame "Arb. plane point" {
                n99 = Array Size(array=w459) -> (size(s)=w458:i32)
                n100 = case shown="Default" w458 {
                  selector: w458 -> [w468 _]
                  tunnel: w465 -> [_ w504]
                  tunnel: w464 -> [_ w502]
                  tunnel: w443 -> [_ _]
                  tunnel: [w469 w497] -> w463
                  tunnel: [w470 w496] -> w462
                  tunnel: w461 -> [w470 w495]
                  tunnel: [_ w494] -> w460
                  tunnel: w459 -> [w469 w492]
                  tunnel: [w468 w483] -> w457
                  tunnel: w456 -> [w467 w490]
                  tunnel: w455 -> [_ w489]
                  tunnel: [w467 w487] -> w454
                  tunnel: w453 -> [_ w486]
                  tunnel: w452 -> [_ w481]
                  tunnel: w451 -> [_ w482]
                  tunnel: w450 -> [_ w479]
                  tunnel: w449 -> [_ w477]
                  tunnel: w448 -> [_ w476]
                  tunnel: w447 -> [_ w475]
                  tunnel: w446 -> [_ w474]
                  tunnel: w445 -> [_ w472]
                  tunnel: w444 -> [_ w471]
                  frame 3.. {
                    # "3 points (or more) already entered"
                  }
                  frame Default {
                    # "WARNING!\nComposite ID is not updated correctly\nbut it currently does not matter."
                    # "WARNING!\nCalculate the ROI time correctly.\nI am not sure what it would be."
                    # "Less than 3 points"
                    n101 = To Double Precision Float(number=w504) -> (double precision float=w499:dbl[])
                    n102 = Increment(x=w490) -> (x+1=w491:i32)
                    n103 = Select(t=w490, s=w489, f=w491) -> (s? t:f=w487:i32)
                    n104 = Increment(x=w502) -> (x+1=w484:i32)
                    n105 = Index Array(array=w499) -> (element #1=w500:dbl, element #2=w493:dbl)  [unwired: 2 in]
                    n106 = To Double Precision Float(number=w477) -> (double precision float=w478:dbl)
                    n107 = To Double Precision Float(number=w484) -> (double precision float=w498:dbl)
                    n108 = To Double Precision Float(number=w487) -> (double precision float=w488:dbl)
                    n109 = Bundle By Name(cluster=T1 {"ROI index"=0.0, "ROI ID"=0.0, "ROI Time (ns)"=0.0, "Pixels in ROI"=0.0, "X start"=0.0, "Y start"=0.0, "Z start"=0.0, "X stop"=0.0, "Y stop"=0.0, "Z stop"=0.0, "Angle (deg)"=0.0, "Composite ID"=0.0, "Number of lines"=0.0, "Frame Size"=0.0, "Zoom"=0.0, "Laser Power (%)"=0.0, "ROI group ID"=0.0, "Resolution"=0.0, "Dwell Time per pixel"=0.0, "Pixels per miniscan"=0.0, "Original FOV (um)"=0.0, "Apparent Frame Size"=0.0, "Z Plane Idx"=[], "Z Plane codes"=[]} ("X-Y-Z coordinates"), "ROI index"=w498, "ROI ID"=w486, "ROI Time (ns)"=-1.0, "Pixels in ROI"=-1.0 ("#Pixels"), "X start"=w500, "Y start"=w493, "X stop"=w500, "Y stop"=w493, "Z Plane Idx"=w481, "Z Plane codes"=w482, "Composite ID"=w488, "Z start"=w479, "Z stop"=w479, "Frame Size"=w478, "Zoom"=w476, "Resolution"=w475, "Dwell Time per pixel"=w474, "Original FOV (um)"=w472, "Laser Power (%)"=w471) -> (w503:T1)
                    n110 = call "Prevent over max lines.vi"("Existing number of lines across all ROI"=w495, "Array in"=w492, "X-Y-Z coordinates"=w503, "New number of lines to be added (1)"=1, "Number of ROI"=w484) -> ("Resulting number of lines across all ROI"=w496:i32, "Array out"=w497:T1[], "Exceeded 1024 lines"=w494:bool, "Number of ROI"=w483:i32)  [unwired: 5 in, 2 out]
                  }
                }
              }
              frame "MiniScan" {
                n111 = To Double Precision Float(number=w516) -> (double precision float=w511:dbl)
                n112 = To Double Precision Float(number=w528) -> (double precision float=w541:dbl[])
                n113 = Increment(x=w543) -> (x+1=w523:i32)
                n114 = Index Array(array=w541) -> (element #1=w525:dbl, element #2=w542:dbl, element #3=w535:dbl, element #4=w538:dbl)  [unwired: 4 in]
                n115 = Multiply(x=w511, y=w510) -> (x*y=w507:dbl)
                n116 = call "Calculate angle.vi"("XY Coordinates"=w528) -> ("Angle (deg)"=w526:dbl)  [unwired: 10 in]
                n117 = call "Calculate miniscan pixels XY only.vi"("Resolution multiplier"=w524, "XY Coordinates (zero based)"=w528) -> ("Pixels in ROI"=w527:dbl, "X pixels"=w512:dbl)  [unwired: 7 in, 1 out]
                n118 = Divide(x=w508, y=w507) -> (x/y=w509:dbl)
                n119 = To Double Precision Float(number=w523) -> (double precision float=w539:dbl)
                n120 = Multiply(x=w540, y=w527) -> (x*y=w505:dbl)
                n121 = Bundle By Name(cluster=T1 {"ROI index"=0.0, "ROI ID"=0.0, "ROI Time (ns)"=0.0, "Pixels in ROI"=0.0, "X start"=0.0, "Y start"=0.0, "Z start"=0.0, "X stop"=0.0, "Y stop"=0.0, "Z stop"=0.0, "Angle (deg)"=0.0, "Composite ID"=0.0, "Number of lines"=0.0, "Frame Size"=0.0, "Zoom"=0.0, "Laser Power (%)"=0.0, "ROI group ID"=0.0, "Resolution"=0.0, "Dwell Time per pixel"=0.0, "Pixels per miniscan"=0.0, "Original FOV (um)"=0.0, "Apparent Frame Size"=0.0, "Z Plane Idx"=[], "Z Plane codes"=[]} ("X-Y-Z coordinates"), "Angle (deg)"=w526, "ROI index"=w539, "ROI ID"=w537, "ROI Time (ns)"=w505, "Pixels in ROI"=w527, "X start"=w525, "Y start"=w542, "X stop"=w535, "Y stop"=w538, "Number of lines"=1.0, "Z Plane Idx"=w520, "Z Plane codes"=w521, "Z start"=w517, "Z stop"=w517, "Frame Size"=w511, "Zoom"=w515, "Resolution"=w509, "Dwell Time per pixel"=w514, "Pixels per miniscan"=w512, "Original FOV (um)"=w508, "Apparent Frame Size"=w507, "Laser Power (%)"=w506) -> (w533:T1)
                n122 = call "Prevent over max lines.vi"("Existing number of lines across all ROI"=w531, "Array in"=w534, "X-Y-Z coordinates"=w533, "New number of lines to be added (1)"=1, "Number of ROI"=w523) -> ("Resulting number of lines across all ROI"=w530:i32, "Array out"=w532:T1[], "Exceeded 1024 lines"=w529:bool, "Number of ROI"=w522:i32)  [unwired: 5 in, 2 out]
              }
              frame "Comp. MiniScan" {
                # "This case of composite miniscans is currently not in use."
                # "Warning!\nReviewe this wire connection"
                # "Note: this is the time for the miniscan\nsection rather than the total miniscan time."
                n123 = To Double Precision Float(number=w564) -> (double precision float=w582:dbl[])
                n124 = Increment(x=w571) -> (x+1=w574:i32)
                n125 = Index Array(array=w582) -> (element #1=w579:dbl, element #2=w583:dbl, element #3=w578:dbl, element #4=w577:dbl)  [unwired: 4 in]
                n126 = Select(t=w571, s=w573, f=w574) -> (s? t:f=w572:i32)
                n127 = call "Calculate angle.vi"("XY Coordinates"=w564) -> ("Angle (deg)"=w562:dbl)  [unwired: 10 in]
                n128 = call "Calculate rectangle pixels and lines.vi"("No of Z planes"=1, "Resolution multiplier"=w561, "XY Coordinates (zero based)"=w564) -> ("Number of lines (scaled)"=w560:dbl, "Pixels in ROI"=w563:dbl)  [unwired: 6 in, 1 out]
                n129 = Increment(x=w584) -> (x+1=w559:i32)
                n130 = To Double Precision Float(number=w559) -> (double precision float=w580:dbl)
                n131 = Multiply(x=w581, y=w563) -> (x*y=w545:dbl)
                n132 = To Double Precision Float(number=w572) -> (double precision float=w575:dbl)
                n133 = To Double Precision Float(number=w552) -> (double precision float=w553:dbl)
                n134 = Bundle By Name(cluster=T1 {"ROI index"=0.0, "ROI ID"=0.0, "ROI Time (ns)"=0.0, "Pixels in ROI"=0.0, "X start"=0.0, "Y start"=0.0, "Z start"=0.0, "X stop"=0.0, "Y stop"=0.0, "Z stop"=0.0, "Angle (deg)"=0.0, "Composite ID"=0.0, "Number of lines"=0.0, "Frame Size"=0.0, "Zoom"=0.0, "Laser Power (%)"=0.0, "ROI group ID"=0.0, "Resolution"=0.0, "Dwell Time per pixel"=0.0, "Pixels per miniscan"=0.0, "Original FOV (um)"=0.0, "Apparent Frame Size"=0.0, "Z Plane Idx"=[], "Z Plane codes"=[]} ("X-Y-Z coordinates"), "Angle (deg)"=w562, "ROI index"=w580, "ROI ID"=w576, "ROI Time (ns)"=w545, "Pixels in ROI"=w563, "X start"=w579, "Y start"=w583, "X stop"=w578, "Y stop"=w577, "Composite ID"=w575, "Number of lines"=w560, "Z Plane Idx"=w556, "Z Plane codes"=w557, "Z start"=w554, "Z stop"=w554, "Frame Size"=w553, "Zoom"=w551, "Resolution"=w550, "Dwell Time per pixel"=w549, "Original FOV (um)"=w547, "Laser Power (%)"=w546) -> (w569:T1)
                n135 = call "Prevent over max lines.vi"("Existing number of lines across all ROI"=w566, "Array in"=w570, "X-Y-Z coordinates"=w569, "Number of ROI"=w559) -> ("Resulting number of lines across all ROI"=w567:i32, "Array out"=w568:T1[], "Exceeded 1024 lines"=w565:bool, "Number of ROI"=w558:i32)  [unwired: 6 in, 2 out]
              }
              frame "Rectangle" {
                # "Warning->>"
                n136 = To Double Precision Float(number=w594) -> (double precision float=w593:dbl)
                n137 = To Double Precision Float(number=w608) -> (double precision float=w625:dbl[])
                n138 = Array Size(array=w601) -> (size(s)=w600:i32)
                n139 = Index Array(array=w625) -> (element #1=w615:dbl, element #2=w610:dbl, element #3=w614:dbl, element #4=w613:dbl)  [unwired: 4 in]
                n140 = call "Calculate angle.vi"("XY Coordinates"=w608) -> ("Angle (deg)"=w607:dbl)  [unwired: 10 in]
                n141 = call "Calculate rectangle pixels and lines.vi"("No of Z planes"=w600, "Resolution multiplier"=w595, "XY Coordinates (zero based)"=w608) -> ("Number of lines (scaled)"=w611:dbl, "Pixels in ROI"=w612:dbl, "X pixels"=w596:dbl)  [unwired: 6 in]
                n142 = Multiply(x=w593, y=w588) -> (x*y=w590:dbl)
                n143 = Divide(x=w591, y=w590) -> (x/y=w589:dbl)
                n144 = Increment(x=w626) -> (x+1=w604:i32)
                n145 = To Long Integer(number=w611) -> (32bit integer=w605:i32)
                n146 = To Double Precision Float(number=w604) -> (double precision float=w623:dbl)
                n147 = Multiply(x=w609, y=w612) -> (x*y=w586:dbl)
                n148 = Bundle By Name(cluster=T1 {"ROI index"=0.0, "ROI ID"=0.0, "ROI Time (ns)"=0.0, "Pixels in ROI"=0.0, "X start"=0.0, "Y start"=0.0, "Z start"=0.0, "X stop"=0.0, "Y stop"=0.0, "Z stop"=0.0, "Angle (deg)"=0.0, "Composite ID"=0.0, "Number of lines"=0.0, "Frame Size"=0.0, "Zoom"=0.0, "Laser Power (%)"=0.0, "ROI group ID"=0.0, "Resolution"=0.0, "Dwell Time per pixel"=0.0, "Pixels per miniscan"=0.0, "Original FOV (um)"=0.0, "Apparent Frame Size"=0.0, "Z Plane Idx"=[], "Z Plane codes"=[]} ("X-Y-Z coordinates"), "Z Plane Idx"=w601, "Z Plane codes"=w602, "Angle (deg)"=w607, "ROI index"=w623, "ROI ID"=w624, "ROI Time (ns)"=w586, "Pixels in ROI"=w612, "X start"=w615, "Y start"=w610, "X stop"=w614, "Y stop"=w613, "Number of lines"=w611, "Composite ID"=0.0, "Z start"=w599, "Z stop"=w599, "Frame Size"=w593, "Zoom"=w592, "Resolution"=w589, "Dwell Time per pixel"=w597, "Pixels per miniscan"=w596, "Original FOV (um)"=w591, "Apparent Frame Size"=w590, "Laser Power (%)"=w587) -> (w620:T1)
                n149 = call "Prevent over max lines.vi"("Existing number of lines across all ROI"=w617, "Array in"=w621, "X-Y-Z coordinates"=w620, "New number of lines to be added (1)"=w605, "Number of ROI"=w604) -> ("Resulting number of lines across all ROI"=w618:i32, "Array out"=w619:T1[], "Exceeded 1024 lines"=w616:bool, "Number of ROI"=w603:i32)  [unwired: 5 in, 2 out]
              }
              frame "Comp. volume" {
                # "Note: this is the time it takes to scan a single plane rather than the total volume scan time."
                n150 = To Double Precision Float(number=w647) -> (double precision float=w663:dbl[])
                n151 = Increment(x=w668) -> (x+1=w642:i32)
                n152 = Increment(x=w657) -> (x+1=w656:i32)
                n153 = To Double Precision Float(number=w642) -> (double precision float=w661:dbl)
                n154 = Index Array(array=w663) -> (element #1=w664:dbl, element #2=w667:dbl, element #3=w666:dbl, element #4=w665:dbl)  [unwired: 4 in]
                n155 = Select(t=w657, s=w658, f=w656) -> (s? t:f=w655:i32)
                n156 = call "Calculate angle.vi"("XY Coordinates"=w647) -> ("Angle (deg)"=w646:dbl)  [unwired: 10 in]
                n157 = call "Calculate rectangle pixels and lines.vi"("No of Z planes"=1, "Resolution multiplier"=w643, "XY Coordinates (zero based)"=w647) -> ("Number of lines (scaled)"=w644:dbl, "Pixels in ROI"=w645:dbl)  [unwired: 6 in, 1 out]
                n158 = To Double Precision Float(number=w655) -> (double precision float=w659:dbl)
                n159 = To Double Precision Float(number=w634) -> (double precision float=w635:dbl)
                n160 = Multiply(x=w660, y=w645) -> (x*y=w628:dbl)
                n161 = To Long Integer(number=w644) -> (32bit integer=w649:i32)
                n162 = Bundle By Name(cluster=T1 {"ROI index"=0.0, "ROI ID"=0.0, "ROI Time (ns)"=0.0, "Pixels in ROI"=0.0, "X start"=0.0, "Y start"=0.0, "Z start"=0.0, "X stop"=0.0, "Y stop"=0.0, "Z stop"=0.0, "Angle (deg)"=0.0, "Composite ID"=0.0, "Number of lines"=0.0, "Frame Size"=0.0, "Zoom"=0.0, "Laser Power (%)"=0.0, "ROI group ID"=0.0, "Resolution"=0.0, "Dwell Time per pixel"=0.0, "Pixels per miniscan"=0.0, "Original FOV (um)"=0.0, "Apparent Frame Size"=0.0, "Z Plane Idx"=[], "Z Plane codes"=[]} ("X-Y-Z coordinates"), "Angle (deg)"=w646, "ROI index"=w661, "ROI ID"=w662, "ROI Time (ns)"=w628, "Pixels in ROI"=w645, "X start"=w664, "Y start"=w667, "X stop"=w666, "Y stop"=w665, "Z Plane Idx"=w639, "Z Plane codes"=w640, "Number of lines"=w644, "Composite ID"=w659, "Z start"=w637, "Z stop"=w637, "Frame Size"=w635, "Zoom"=w633, "Resolution"=w632, "Dwell Time per pixel"=w631, "Original FOV (um)"=w630, "Laser Power (%)"=w629) -> (w653:T1)
                n163 = call "Prevent over max lines.vi"("Existing number of lines across all ROI"=w650, "Array in"=w654, "X-Y-Z coordinates"=w653, "New number of lines to be added (1)"=w649, "Number of ROI"=w642) -> ("Resulting number of lines across all ROI"=w651:i32, "Array out"=w652:T1[], "Exceeded 1024 lines"=w648:bool, "Number of ROI"=w641:i32)  [unwired: 5 in, 2 out]
              }
            }
            n164 = Add(x=w372, y=w374) -> (x+y=w375:dbl)
          }
          frame "Update ROIs time" {
            n165 = call "Update ROI times.vi"("ROI setup in"=w672) -> ("ROI setup out"=w676:T1[])  [unwired: 10 in]
          }
          frame "Reload last ROI set" {
            # "Reloads the last loaded ROI set, if one was loaded since the ROI Entry screen was called. This allows to easily reset any ROI offsets applied without the need to browse to the loaded ROI file and load it over again."
            n166 = global read "gl_ROI Entry UI globals.vi" "Loaded ROI setup"() -> (w680:T1[])
            n167 = Empty Array?(array=w680) -> (empty?=w682:bool)
            n168 = Select(t=w681, s=w682, f=w680) -> (s? t:f=w679:T1[])
            n169 = for {
              tunnel: w679 -> [w688] mode=indexing
              tunnel: [w687] -> w678 mode=indexing
              n170 = Unbundle By Name(w688) -> ("ROI Time (ns)"=w687:dbl)
            }
            n171 = Add Array Elements(numeric array=w678) -> (sum=w677:dbl)
          }
          frame "Clear Last" {
            n172 = while {
              tunnel: w697 -> [w709]
              tunnel: [w708] -> w696
              shift-right: [w712] -> w700
              shift-left: w695 -> [w706]
              shift-right: [w711] -> w699
              shift-left: w694 -> [w705]
              shift-right: [w703] -> w691
              shift-left: w693 -> [w704]
              shift-right: [w701] -> w689
              shift-left: w690 -> [w702]
              stop <- w707 stop-if-true
              n173 = Greater Than 0?(x=w706) -> (x > 0?=w710:bool)
              n174 = case shown="True" w710 {
                tunnel: [0 w734] -> w712
                tunnel: w705 -> [w717 w737]
                tunnel: [w717 w728] -> w711
                tunnel: w706 -> [_ w736]
                tunnel: w709 -> [w716 w731]
                tunnel: [w716 w730] -> w708
                tunnel: [TRUE w729] -> w707
                tunnel: w704 -> [_ w727]
                tunnel: [0 w726] -> w703
                tunnel: w702 -> [w713 w721]
                tunnel: [w713 w719] -> w701
                frame False {
                  # "No ROIs available"
                }
                frame True {
                  # "ROIs available"
                  n175 = Decrement(x=w736) -> (x-1=w734:i32)
                  n176 = Delete From Array "Delete From Array"(array=w737, length=1, index=w734) -> (deleted portion=w733:T1[], array with subset deleted=w728:T1[])
                  n177 = Index Array(array=w733) -> (element=w722:T1)  [unwired: 1 in]
                  n178 = Unbundle By Name(w722) -> ("ROI ID"=w732:dbl)
                  n179 = Unbundle By Name(w722) -> ("ROI Time (ns)"=w720:dbl)
                  n180 = To Unsigned Word Integer(number=w732) -> (unsigned 16bit integer=w725:u16)
                  n181 = Type Cast(type=ROI_ID_Enum."Point" ("ROI Type"), x=w725) -> (*(type *) &x=w724:T4)
                  n182 = Subtract(x=w721, y=w720) -> (x-y=w719:dbl)
                  n183 = case shown="\"Comp. volume\"" w724 {
                    tunnel: w731 -> [w741 w745 w752 w760 w780]
                    tunnel: [w741 w745 w752 w759 w779] -> w730
                    tunnel: [TRUE TRUE TRUE w756 w776] -> w729
                    tunnel: w728 -> [_ _ _ w755 w775]
                    tunnel: w722 -> [_ _ _ w758 w778]
                    tunnel: w727 -> [w739 w743 w748 w754 w772]
                    tunnel: [w738 w742 w747 w753 w771] -> w726
                    tunnel: w722 -> [_ _ w746 _ w770]
                    frame "Point", Default {
                      # "Not a composite"
                      n184 = Decrement(x=w739) -> (x-1=w738:i32)
                    }
                    frame "MiniScan" {
                      # "Not a composite"
                      n185 = Decrement(x=w743) -> (x-1=w742:i32)
                    }
                    frame "Rectangle" {
                      # "Not a composite"
                      n186 = Unbundle By Name(w746) -> ("Number of lines"=w749:dbl)
                      n187 = To Long Integer(number=w749) -> (32bit integer=w750:i32)
                      n188 = Subtract(x=w748, y=w750) -> (x-y=w747:i32)
                    }
                    frame "Comp. MiniScan" {
                      # "Composite mscn, or volume"
                      n189 = Array Size(array=w755) -> (size(s)=w757:i32)
                      n190 = Decrement(x=w760) -> (x-1=w759:i32)
                      n191 = case shown="Default" w757 {
                        selector: w757 -> [_ w763]
                        tunnel: w755 -> [_ w769]
                        tunnel: w758 -> [_ w766]
                        tunnel: [TRUE w762] -> w756
                        frame 0 {
                          # "No more ROIs left"
                        }
                        frame Default {
                          # "Checks if the previous ROI \nbelongs to the same composite. If it does, then keeps the loop going, until all component ROIs have been removed (i.e. an entire volume ROI removed)."
                          # "Previous"
                          # "Current"
                          # "No more ROIs available"
                          n192 = Decrement(x=w763) -> (x-1=w768:i32)
                          n193 = Index Array(array=w769, index=w768) -> (element=w767:T1)
                          n194 = Unbundle By Name(w767) -> ("Composite ID"=w765:dbl)
                          n195 = Unbundle By Name(w766) -> ("Composite ID"=w764:dbl)
                          n196 = Not Equal?(x=w765, y=w764) -> (x != y?=w762:bool)
                        }
                      }
                      n197 = Decrement(x=w754) -> (x-1=w753:i32)
                    }
                    frame "Comp. volume" {
                      # "Composite mscn, or volume"
                      n198 = Unbundle By Name(w770) -> ("Number of lines"=w773:dbl)
                      n199 = Array Size(array=w775) -> (size(s)=w777:i32)
                      n200 = case shown="Default" w777 {
                        selector: w777 -> [_ w783]
                        tunnel: w775 -> [_ w789]
                        tunnel: w778 -> [_ w786]
                        tunnel: [TRUE w782] -> w776
                        frame 0 {
                          # "No more ROIs left"
                        }
                        frame Default {
                          # "Checks if the previous ROI \nbelongs to the same composite. If it does, then keeps the loop going, until all component ROIs have been removed (i.e. an entire volume ROI removed)."
                          # "Previous"
                          # "Current"
                          # "No more ROIs available"
                          n201 = Decrement(x=w783) -> (x-1=w788:i32)
                          n202 = Index Array(array=w789, index=w788) -> (element=w787:T1)
                          n203 = Unbundle By Name(w787) -> ("Composite ID"=w785:dbl)
                          n204 = Unbundle By Name(w786) -> ("Composite ID"=w784:dbl)
                          n205 = Not Equal?(x=w785, y=w784) -> (x != y?=w782:bool)
                        }
                      }
                      n206 = Decrement(x=w780) -> (x-1=w779:i32)
                      n207 = To Long Integer(number=w773) -> (32bit integer=w774:i32)
                      n208 = Subtract(x=w772, y=w774) -> (x-y=w771:i32)
                    }
                  }
                }
              }
            }
          }
          frame "Clear All" {
          }
          frame "Offset all ROI", "Offset visible ROI" {
            n209 = call "ROI entry-Offset ROI (core).vi"("Function"=w798, "ROI setup in"=w802, "Offsets cluster in"=w800) -> ("ROI setup"=w799:T1[])  [unwired: 8 in]
          }
          frame "Delete ROI" {
            n210 = call "ROI entry screen-Delete ROIs.vi"("No of lines I/p"=w811, "ROI Time (ns)"=w807, "Deletion Idx"="ROIs for deletion", "ROI setup I/P"=w815) -> ("ROI Time (ns)o/p"=w806:dbl, "No of ROIs"=w813:i32, "ROI setup O/P"=w814:T1[], "No of lines o/p"=w810:i32)  [unwired: 4 in]
          }
          frame "Modify ROI Parameters" {
            # "NOT IN USE"
            n211 = Index Array(array=w817, index="ROI Setup Array Idx to modify") -> (element=w829:T1)
            n212 = call "Prevent over max lines.vi"("Existing number of lines across all ROI"=w821, "Modify"=TRUE, "Array in"=w817, "Mod. ROI Idx"="ROI Setup Array Idx to modify", "X-Y-Z coordinates"="XYZ", "Number of ROI"=w819) -> ("Resulting number of lines across all ROI"=w820:i32, "Array out"=w825:T1[], "Modified/Added"=w816:bool, "Number of ROI"=w818:i32)  [unwired: 4 in, 2 out]
            n213 = Unbundle By Name("XYZ") -> ("ROI Time (ns)"=w827:dbl)
            n214 = case shown="True" w816 {
              tunnel: w829 -> [_ w838]
              tunnel: w828 -> [w832 w837]
              tunnel: w827 -> [_ w834]
              tunnel: [w832 w833] -> w826
              frame False {
              }
              frame True {
                n215 = Unbundle By Name(w838) -> ("ROI Time (ns)"=w836:dbl)
                n216 = Subtract(x=w837, y=w836) -> (x-y=w835:dbl)
                n217 = Add(x=w835, y=w834) -> (x+y=w833:dbl)
              }
            }
          }
          frame "Modify Dwell Time" {
            n218 = for {
              tunnel: w847 -> [w853] mode=indexing
              tunnel: "Dwell Time [us]" -> [w848]
              tunnel: [w854] -> w845 mode=indexing
              tunnel: [w851] -> w840 mode=indexing
              n219 = Unbundle By Name(w853) -> ("Pixels in ROI"=w852:dbl)
              n220 = Multiply(x=w848, y=1000.0) -> (x*y=w849:dbl)
              n221 = Multiply(x=w849, y=w852) -> (x*y=w851:dbl)
              n222 = Bundle By Name(cluster=w853, "Dwell Time per pixel"=w848, "ROI Time (ns)"=w851) -> (w854:T1)
            }
            n223 = Add Array Elements(numeric array=w840) -> (sum=w839:dbl)
          }
          frame "Modify Laser Power" {
            n224 = for {
              tunnel: w862 -> [w865] mode=indexing
              tunnel: "Laser Power %" -> [w864]
              tunnel: [w863] -> w860 mode=indexing
              n225 = Bundle By Name(cluster=w865, "Laser Power (%)"=w864) -> (w863:T1)
            }
          }
        }
      }
      n226 = global read "General Globals.vi" "Hardware limitation (number of lines across al ROI)"() -> (w27:i32)
      n227 = call "ROI entry-Update number of ROI ind.vi"("error in (no error)"=w25, "ROI Setup"=w24) -> ("error out"=w23:errorcluster)  [unwired: 9 in]
      n228 = Subtract(x=w27, y=w28) -> (x-y=w20:i32)
      n229 = Less Or Equal To 0?(x=w20) -> (x <= 0?=w19:bool)
      n230 = call "ROI entry-Set number of lines left ind.vi"("error in (no error)"=w23, "Number of lines left"=w20) -> ("error out"=w22:errorcluster)  [unwired: 9 in]
    }
    frame Error {
    }
  }
  "error out" <- w14
  "ROI Setup" <- w16
  "Number of ROI" <- w11
  "Last composite ID" <- w10
  "Number of lines left" <- w5
  "Exceeded limit number of lines" <- w4
  "No lines left" <- w2
  "Total ROI time" <- w1
